vi "Off Mode Standby Mode Power Measure SM.vi"(0 "Power":T3={"Yokogawa"={"WT210"={"Sample Rate (1: 0.25s)"=1, "A Range (12: 20A)"=11, "V Range (6: 600V)"=4, "Power VISA Yokogawa WT210"="WT210"}, "WT500"={"Power VISA Yokogawa WT500"="WT500", "V Range (8: 1000V)"=6, "I Range (7: 40A)"=7, "Update Rate (3: 500ms)"=2}, "WT310_2"={"Sample Rate (1: 0.25s)"=1, "A Range (12: 20A)"=11, "V Range (6: 600V)"=4, "Power VISA Yokogawa WT310_2"=""}, "WT310_3"={"Sample Rate (1: 0.25s)"=1, "A Range (12: 20A)"=11, "V Range (6: 600V)"=4, "Power VISA Yokogawa WT310_3"=""}}, "Aplus"={"Aplus IP Address"="192.168.1.101", "Remote Port"=502, "Instrument"="APLUS", "Instr Driver Revision"="1.03.0053"}, "Power Limits"={"Crest Factor"={"Upper Limit"=1.49, "Lower Limit"=1.34}, "Harmonic Content"={"Uthd"=2.0}, "Voltage"={"% Error"=2.0}, "Stability"={"<1 Watt "={"Wattage"=1.0, "Slope (mW/H)"=10.0}, ">1 Watt"={"1%Power/Hour"=1.0}}}, "Nominal Voltage"=120, "Time Limit (s)"=10800.0, "Power Variation Limit (%)"=50.0, "Power Supply"={"Chroma 61605"="CHROMA", "Use Chroma?"=FALSE}} {"Yokogawa"."WT310_3"."V Range (6: 600V)" items=["Auto", "15V", "30V", "60V", "150V", "300V", "600V"]; "Yokogawa"."WT310_3"."A Range (12: 20A)" items=["Auto", "5mA", "10mA", "20mA", "50mA", "100mA", "200mA", "0.5A", "1A", "2A", "5A", "10A", "20A", "50mV", "100mV", "200mV", "2.5V", "5V", "10V"]; "Yokogawa"."WT310_3"."Sample Rate (1: 0.25s)" items=["0.1s", "0.25s", "0.5s", "1s", "2s", "5s"]; "Yokogawa"."WT310_2"."V Range (6: 600V)" items=["Auto", "15V", "30V", "60V", "150V", "300V", "600V"]; "Yokogawa"."WT310_2"."A Range (12: 20A)" items=["Auto", "5mA", "10mA", "20mA", "50mA", "100mA", "200mA", "0.5A", "1A", "2A", "5A", "10A", "20A", "50mV", "100mV", "200mV", "2.5V", "5V", "10V"]; "Yokogawa"."WT310_2"."Sample Rate (1: 0.25s)" items=["0.1s", "0.25s", "0.5s", "1s", "2s", "5s"]; "Yokogawa"."WT500"."Update Rate (3: 500ms)" items=["-", "100ms", "200ms", "500ms", "1s", "2s", "5s"]; "Yokogawa"."WT500"."I Range (7: 40A)" items=["AUTO", "500 mA", "1 A", "2 A", "5 A", "10 A", "20 A", "40 A", "S-AUTO", "50 mV", "100 mV", "200 mV", "500 mV", "1 V", "2 V", "5 V", "10 V", "250 mA", "500 mA", "1 A", "2.5 A", "5 A", "10 A", "20 A", "25 mV", "50 mV", "100 mV", "250 mV", "500 mV", "1 V", "2.5 V", "5 V"]; "Yokogawa"."WT500"."V Range (8: 1000V)" items=["AUTO", "15", "30", "60", "100", "150", "300", "600", "1000", "7.5", "15", "30", "50", "75", "150", "300", "500"]; "Yokogawa"."WT210"."V Range (6: 600V)" items=["Auto", "15V", "30V", "60V", "150V", "300V", "600V"]; "Yokogawa"."WT210"."A Range (12: 20A)" items=["Auto", "5mA", "10mA", "20mA", "50mA", "100mA", "200mA", "0.5A", "1A", "2A", "5A", "10A", "20A", "50mV", "100mV", "200mV", "2.5V", "5V", "10V"]; "Yokogawa"."WT210"."Sample Rate (1: 0.25s)" items=["0.1s", "0.25s", "0.5s", "1s", "2s", "5s"]}, 1 "Station Label":string="Single Phase 2W", 2 "Appliance Common":T1, 5 "Power Analyzer":T4=enum."APLUS", 11 "Error In":errorcluster) -> (6 "Standby Power Out":T5={"Standby Power Spreadsheet"=[], "Standby Power - Pia (Watts)"=0.0, "Off Mode Power - Poff (Watts)"=0.0, "Sia hr/yr"=8620.0, "Soff hr/yr"=0.0, "Yearly Energy Etso kWh/yr"=0.0, "Maximum Power (Watts)"=0.0, "Power Variation (%)"=0.0, "Slope (mW/hr)"=0.0, "Final Harmonics-U1 (%)"="", "Final Harmonics-U2 (%)"="", "Energy (Wh)"=0.0}, 15 "Error Out":errorcluster)   [LabVIEW 2018]
uses:
  Type Definitions/UTILITY Power Inputs Control.ctl
  Type Definitions/UTILITY Power Analyzer.ctl
  Type Definitions/Standby Power Main Data.ctl
  Custom Pallet Controls/Custom Pallet DBL.ctl
  Washer DOE/Type Definitions/DOE Appliance Common.ctl
  Type Definitions/Standby Power Data Arrays.ctl
  Type Definitions/Standby Power Test Routine.ctl
  Drivers/Yokogawa WT200 Series/Yokogawa WT200 Series.lvlib
panel:
  out "User Notice":string
  out "Description 4":string="Single Phase 2W"
  out "Elapsed Time.":dbl format="%<%H:%M:%S>t"
  in  "Disable Plot":bool
  in  "Pause Graph":bool
  out "XY Graph":T2(graph)
  in  "Y-Axis-2":string(combo)
  in  "Y-Axis-1":string(combo)
  in  "X-Axis":string(combo)
  out "Data":string[][](array[string])
  out "Description":string="IEC 62301 Edition 2.0 2011-01\nHousehold Electrical Appliances - Measurment of standby power"
  in  "Tab Control":enum32{"Input Parameters", "Debug"}(tab)
  in  "Debug":bool
  out "Current State":string
  in  "First 1/3 Timer\n(300 Seconds)":dbl=300.0
  in  "Last 2/3 Timer\n(600 Seconds)":dbl=600.0
  in  "Standby Power In":T5={"Standby Power Spreadsheet"=[], "Standby Power - Pia (Watts)"=0.0, "Off Mode Power - Poff (Watts)"=0.0, "Sia hr/yr"=8620.0, "Soff hr/yr"=0.0, "Yearly Energy Etso kWh/yr"=0.0, "Maximum Power (Watts)"=0.0, "Power Variation (%)"=0.0, "Slope (mW/hr)"=0.0, "Final Harmonics-U1 (%)"="", "Final Harmonics-U2 (%)"="", "Energy (Wh)"=0.0}
  in  "Debug?":bool=TRUE
  out "Debug State":string[](array[string])
  out "Initialization File":string[][](array[string])
  in  "K(0.3)":dbl=0.3 format="%#_13g"
  out "Main Loop Rate":T6 format="%.2f"
  in  "Initialize Rate":bool
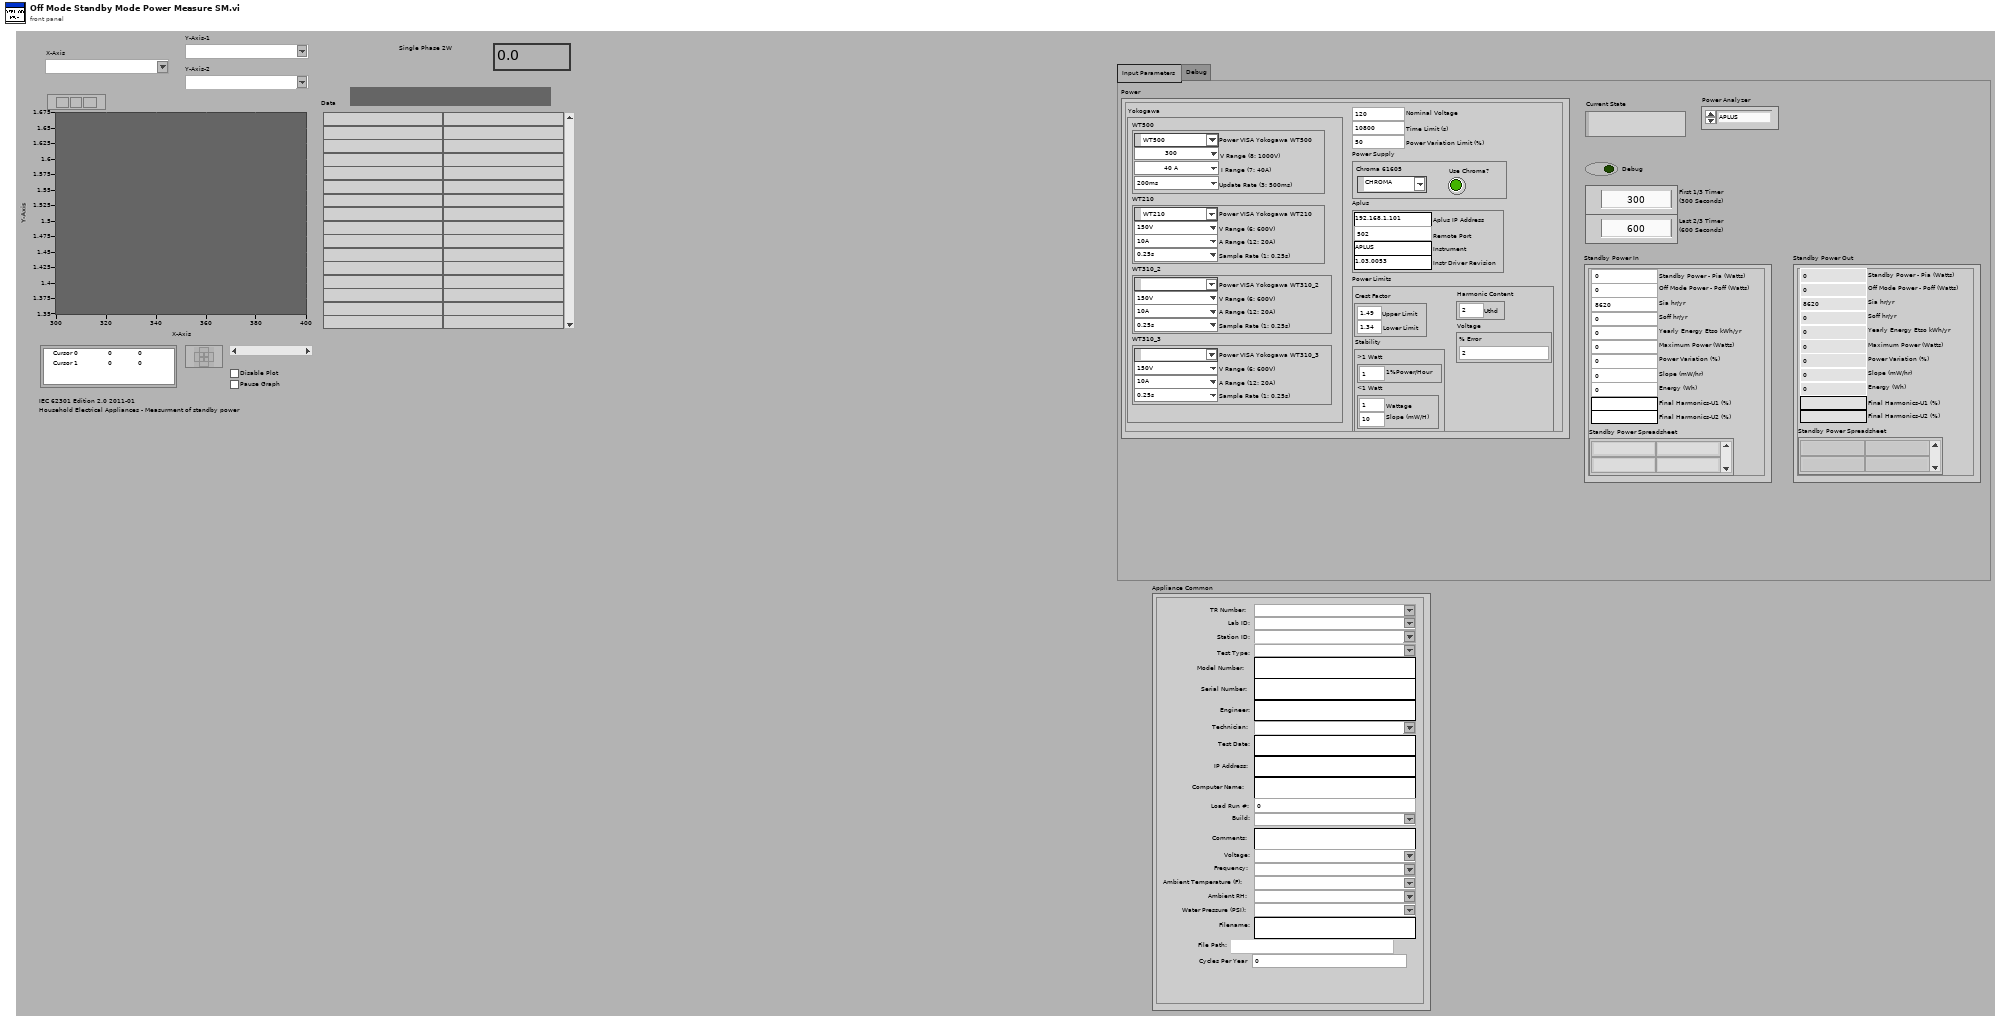
[diagram p1: front panel]
types:
  T1 = typedef "DOE Appliance Common.ctl" = cluster{"Engineer:":string, "Model Number:":string, "Serial Number:":string, "Comments:":string, "Station ID:":string, "Technician:":string, "TR Number:":string, "Lab ID:":string, "Voltage:":string, "Water Pressure (PSI):":string, "Test Date:":string, "Computer Name:":string, "IP Address:":string, "Ambient RH:":string, "Frequency:":string, "Build:":string, "Filename:":string, "Test Type:":string, "Load Run #:":i32, "Ambient Temperature (F):":string, "File Path:":path, "Cycles Per Year":u32}
  T2 = cluster{"Time Array Output":dbl[], "Data Array Output":dbl[]}[]
  T3 = typedef "UTILITY Power Inputs Control.ctl" = cluster{"Yokogawa":cluster{"WT210":cluster{"Sample Rate (1: 0.25s)":i32, "A Range (12: 20A)":i32, "V Range (6: 600V)":i32, "Power VISA Yokogawa WT210":refnum<visa-resource-name>}, "WT500":cluster{"Power VISA Yokogawa WT500":refnum<visa-resource-name>, "V Range (8: 1000V)":i32, "I Range (7: 40A)":i32, "Update Rate (3: 500ms)":i32}, "WT310_2":cluster{"Sample Rate (1: 0.25s)":i32, "A Range (12: 20A)":i32, "V Range (6: 600V)":i32, "Power VISA Yokogawa WT310_2":refnum<visa-resource-name>}, "WT310_3":cluster{"Sample Rate (1: 0.25s)":i32, "A Range (12: 20A)":i32, "V Range (6: 600V)":i32, "Power VISA Yokogawa WT310_3":refnum<visa-resource-name>}}, "Aplus":cluster{"Aplus IP Address":string, "Remote Port":i32, "Instrument":string, "Instr Driver Revision":string}, "Power Limits":cluster{"Crest Factor":cluster{"Upper Limit":dbl, "Lower Limit":dbl}, "Harmonic Content":cluster{"Uthd":dbl}, "Voltage":cluster{"% Error":dbl}, "Stability":cluster{"<1 Watt ":cluster{"Wattage":dbl, "Slope (mW/H)":dbl}, ">1 Watt":cluster{"1%Power/Hour":dbl}}}, "Nominal Voltage":i32, "Time Limit (s)":dbl, "Power Variation Limit (%)":dbl, "Power Supply":cluster{"Chroma 61605":refnum<visa-resource-name>, "Use Chroma?":bool}}
  T4 = typedef "UTILITY Power Analyzer.ctl" = enum16{"", "APLUS", "WT210", "WT500", "WT300", "OSI", "Debug", "WT230", "WT300_1", "WT300_2"}
  T5 = typedef "Standby Power Main Data.ctl" = cluster{"Standby Power Spreadsheet":string[][], "Standby Power - Pia (Watts)":dbl, "Off Mode Power - Poff (Watts)":dbl, "Sia hr/yr":dbl, "Soff hr/yr":dbl, "Yearly Energy Etso kWh/yr":dbl, "Maximum Power (Watts)":dbl, "Power Variation (%)":dbl, "Slope (mW/hr)":dbl, "Final Harmonics-U1 (%)":string, "Final Harmonics-U2 (%)":string, "Energy (Wh)":dbl}
  T6 = typedef "Custom Pallet DBL.ctl" = dbl
  T7 = cluster{"Part 1":bool, "Part 2":bool, "Part 3":bool}
  T8 = enum32{"invalid app kind", "Development System", "Run Time System", "Student Edition", "Embedded LabVIEW", "Evaluation", "Custom"}
  T9 = enum32{"Invalid", "Standard", "Closed", "Hidden", "Minimized", "Maximized"}
  T10 = typedef "Standby Power Data Arrays.ctl" = cluster{"15 Min Data Array":dbl[][], "5 Min Data Array":dbl[][]}
  T11 = typedef "Standby Power Test Routine.ctl" = cluster{"Part 1":bool, "Part 2":bool, "Part 3":bool}
  T12 = cluster{"Core":cluster{"Current VI Reference":refnum<vi>, "Close Panel on Exit?":bool}, "Standby Power Array":T10, "Power ":T3, "Loop Index":i32, "Header File":string[][], "Power Analyzer":T4, "Standby Power In":T5, "Total Array":string[][], "Current State":T11, "Save Data":string[][], "Write Header":bool, "Data Process Timer Reset":bool, "Error?":bool, "Reset Timer?":bool, "Appliance Common":T1}
  T13 = cluster{"Current VI Reference":refnum<vi>, "Close Panel on Exit?":bool}
  T14 = typedef "UTILITY Power Data.ctl" = cluster{"Current (A):Element 1":dbl, "Current (A):Element 2":dbl, "Power (W):Sigma":dbl, "Watt Hours (Wh):Sigma":dbl, "Voltage (V):Element 2":dbl, "Voltage (V):Element 1":dbl, "Current Crest Factor:Element 1":dbl, "Current Crest Factor:Element 2":dbl, "Voltage Harmonic (%):Element 1":dbl, "Voltage Harmonic (%):Element 2":dbl, "Voltage Crest Factor:Element 1":dbl, "Voltage Crest Factor:Element 2":dbl, "Time:Element 1":dbl, "Frequency (Hz):Element 1":dbl, "Apparent Power (VA):Element 1":dbl, "Apparent Power (VA):Element 2":dbl, "Power Factor:Element 1":dbl, "Power Factor:Element 2":dbl, "Max Watt Hours":dbl, "Voltage (V):Element 2 Avg":dbl, "Voltage (V):Element 1 Avg":dbl}
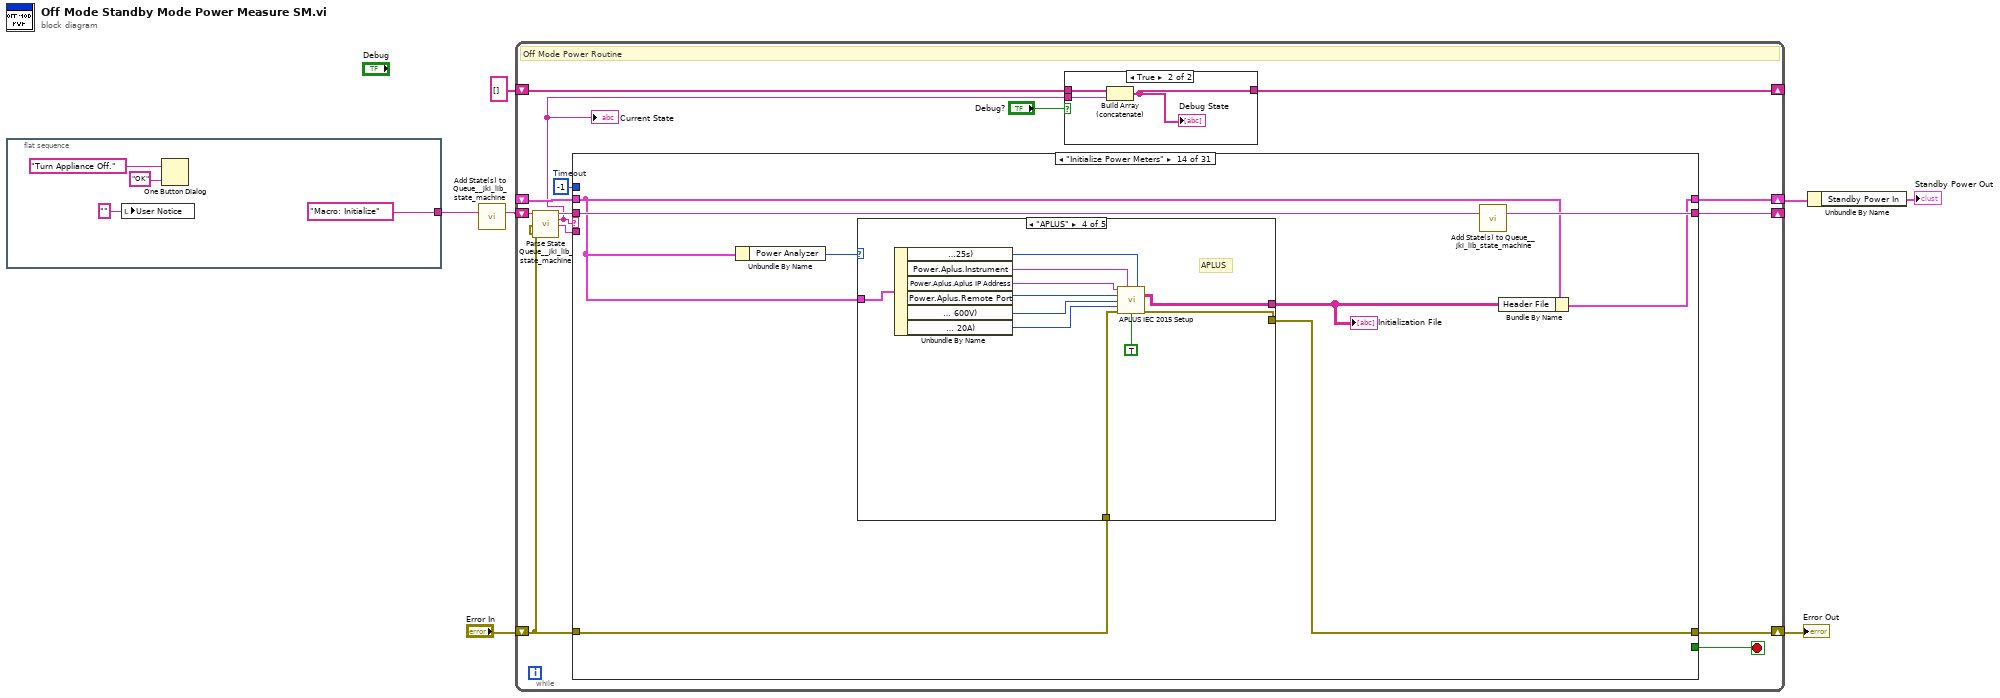
[diagram p0: block diagram]
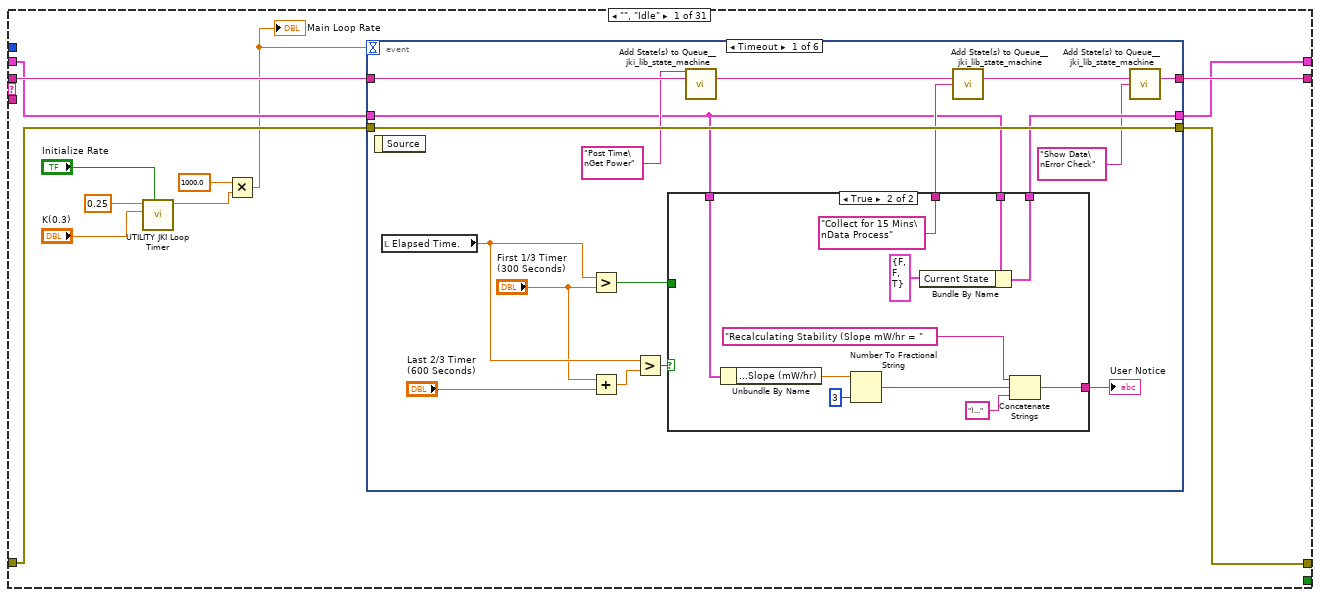
[diagram p3: hidden frame]
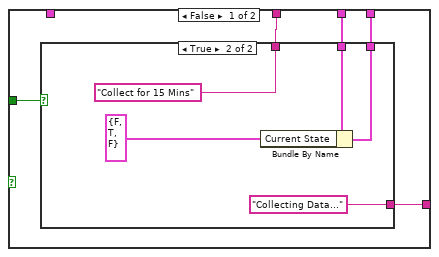
[diagram p4: hidden frame]
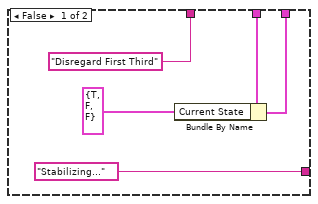
[diagram p5: hidden frame]
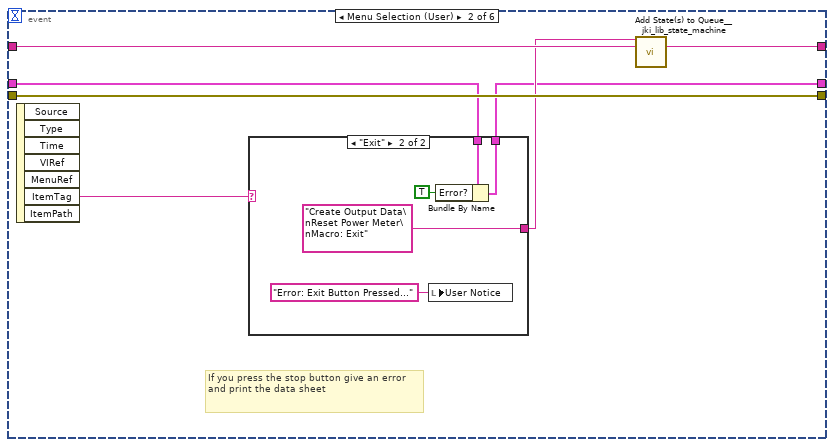
[diagram p6: hidden frame]
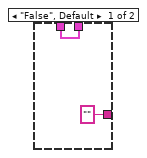
[diagram p7: hidden frame]
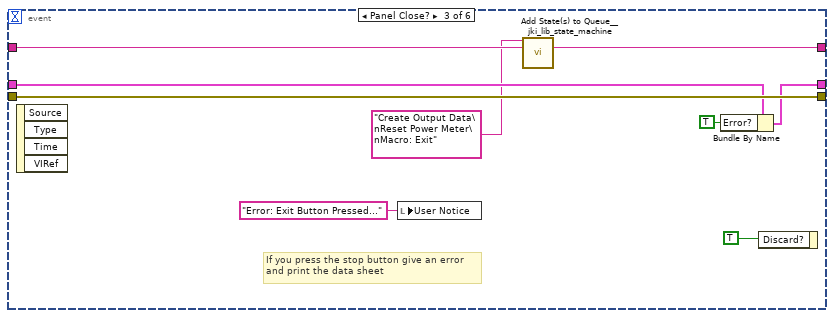
[diagram p8: hidden frame]
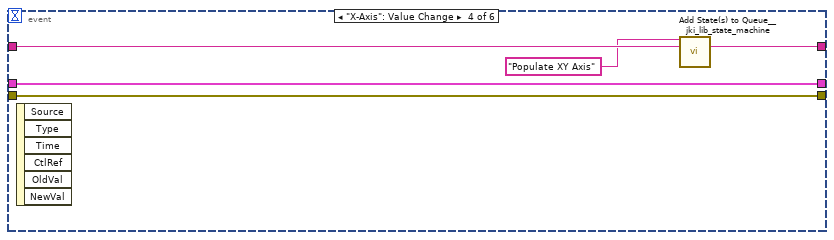
[diagram p9: hidden frame]
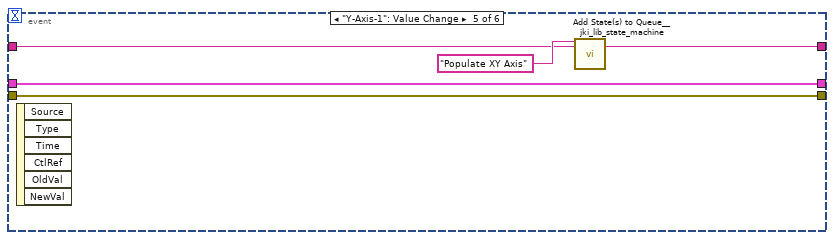
[diagram p10: hidden frame]
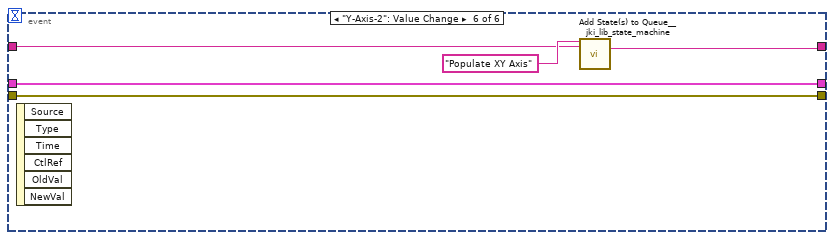
[diagram p11: hidden frame]
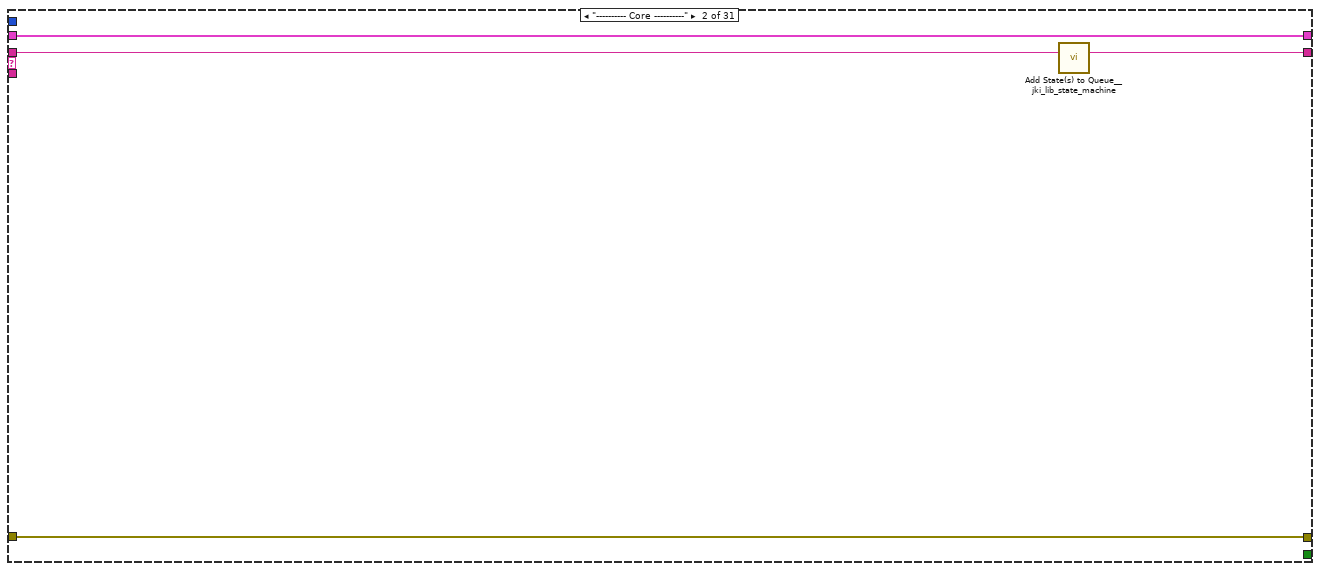
[diagram p12: hidden frame]
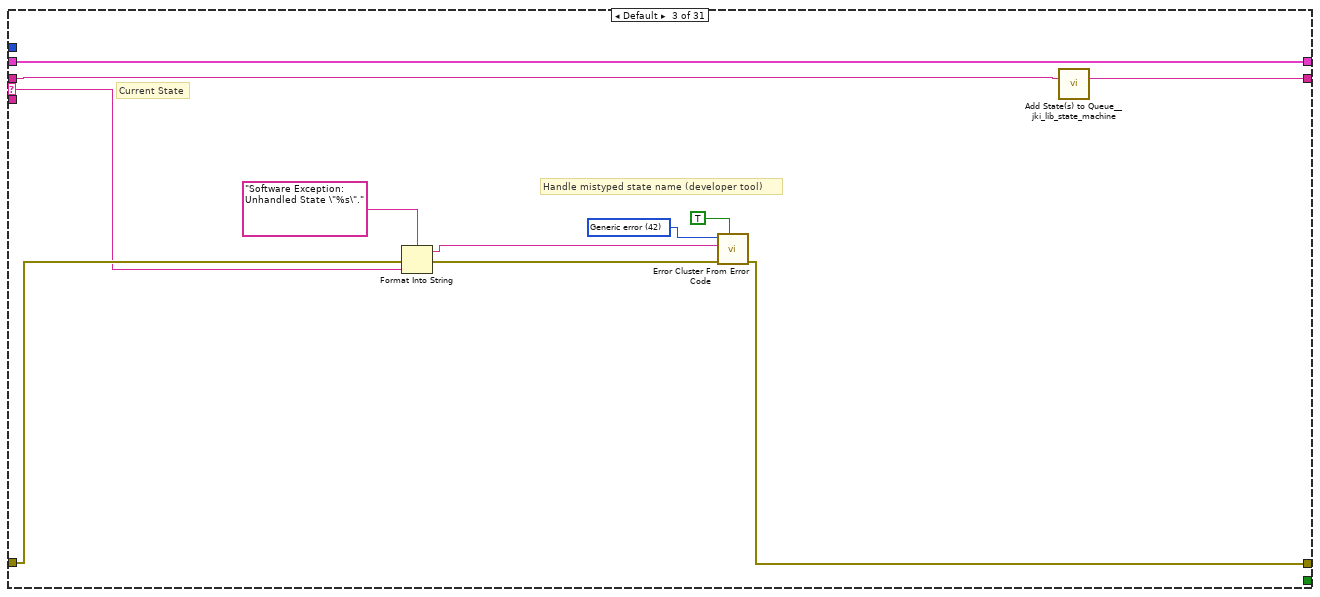
[diagram p13: hidden frame]
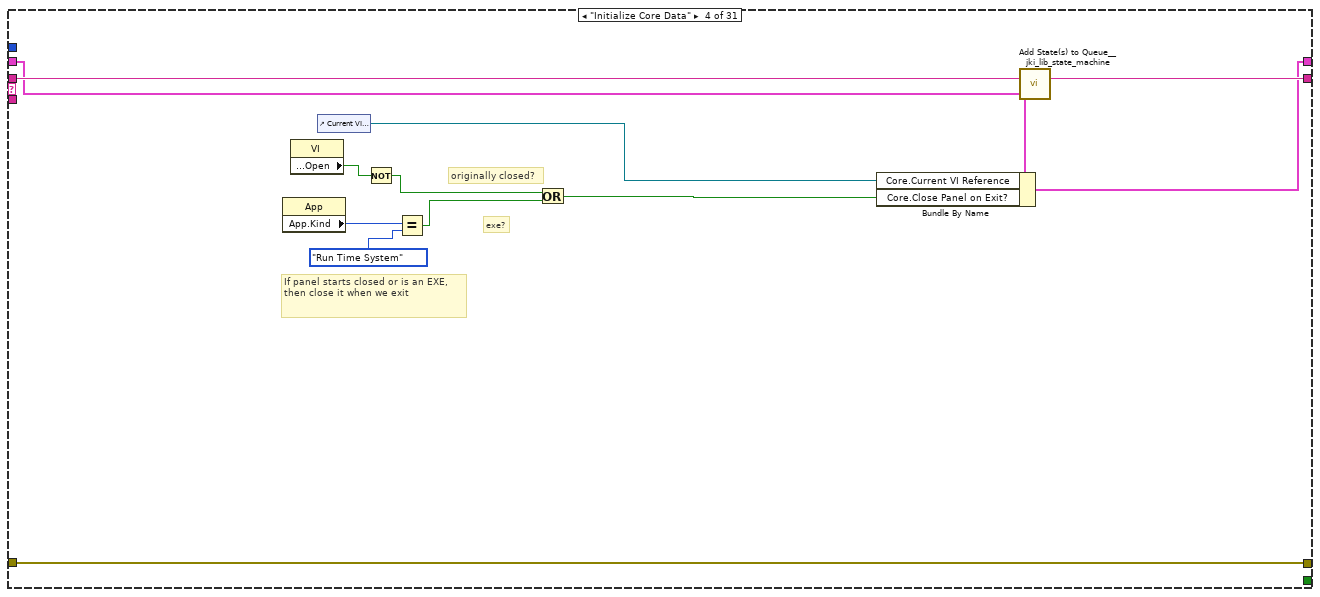
[diagram p14: hidden frame]
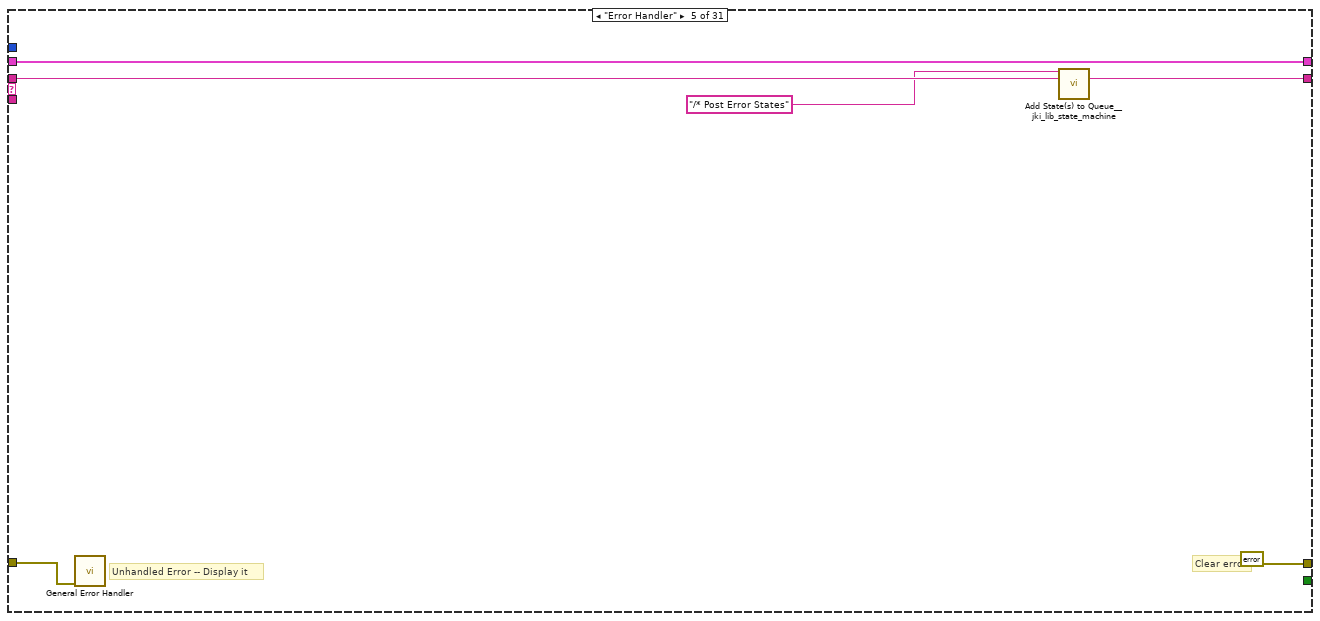
[diagram p15: hidden frame]
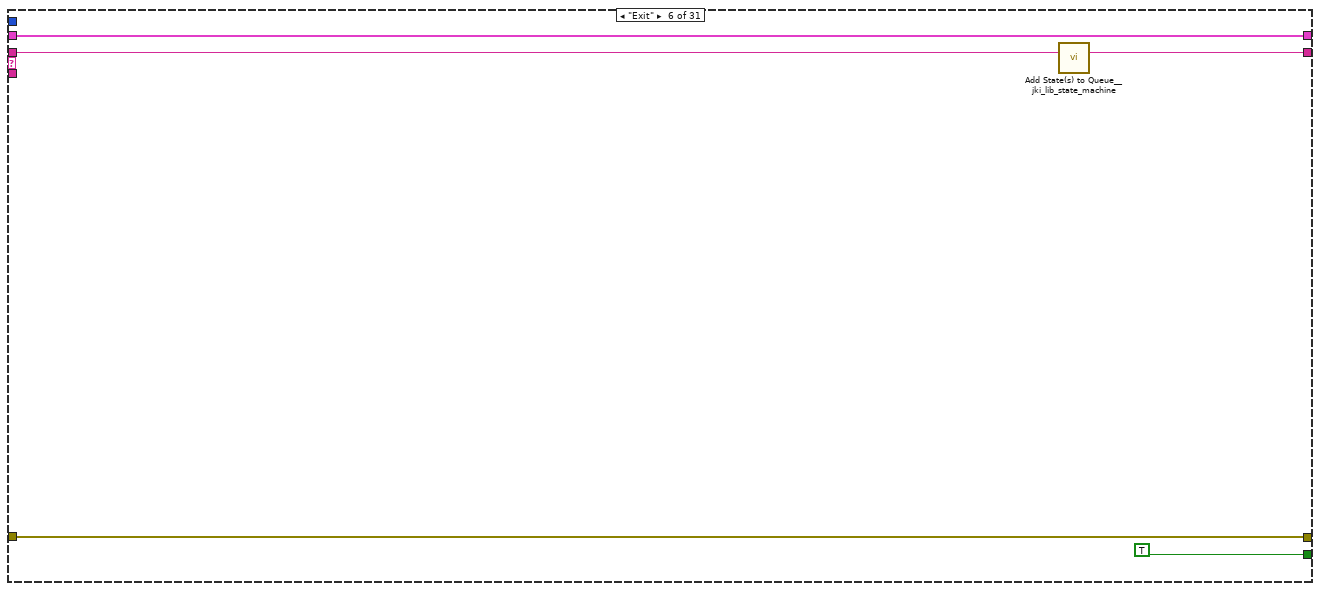
[diagram p16: hidden frame]
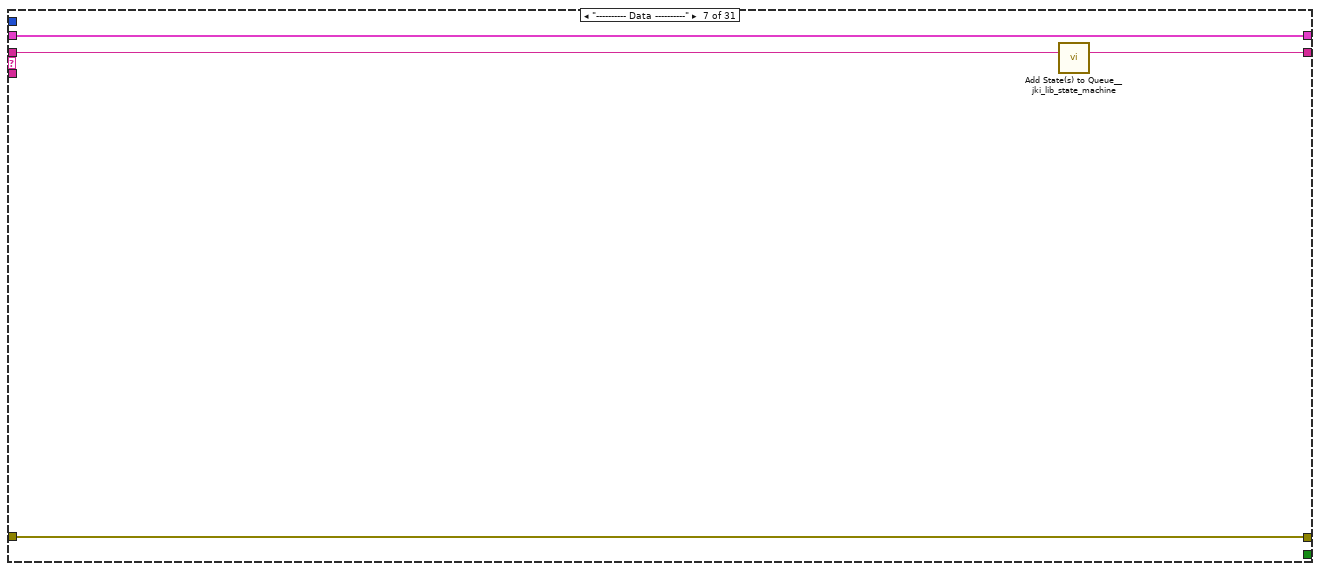
[diagram p17: hidden frame]
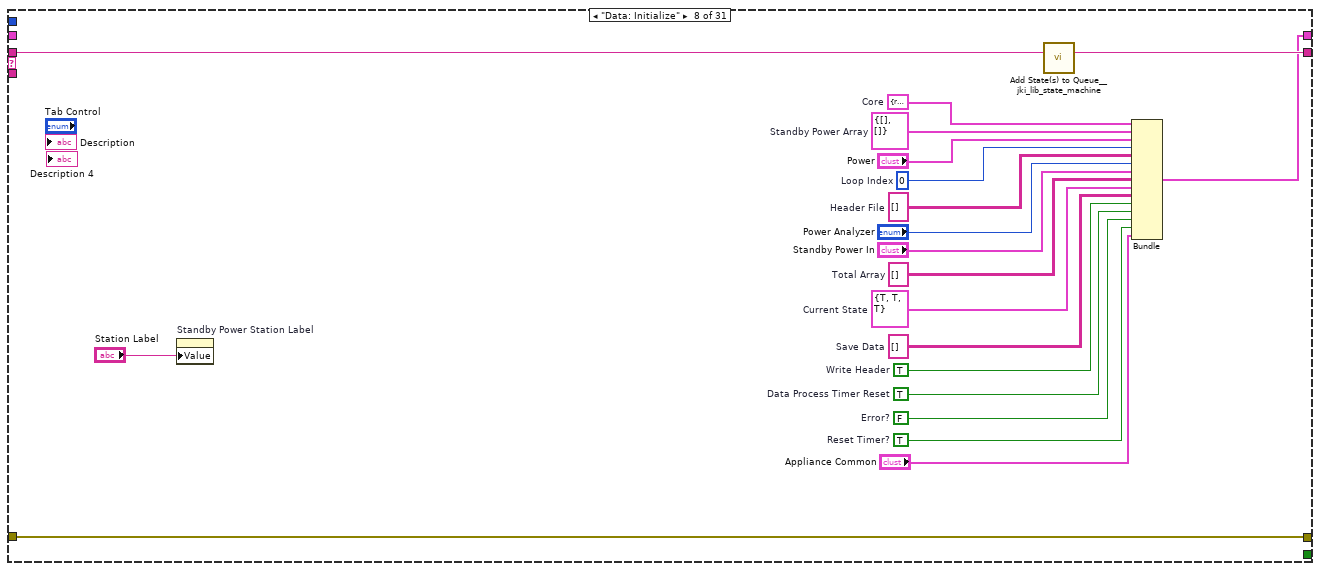
[diagram p18: hidden frame]
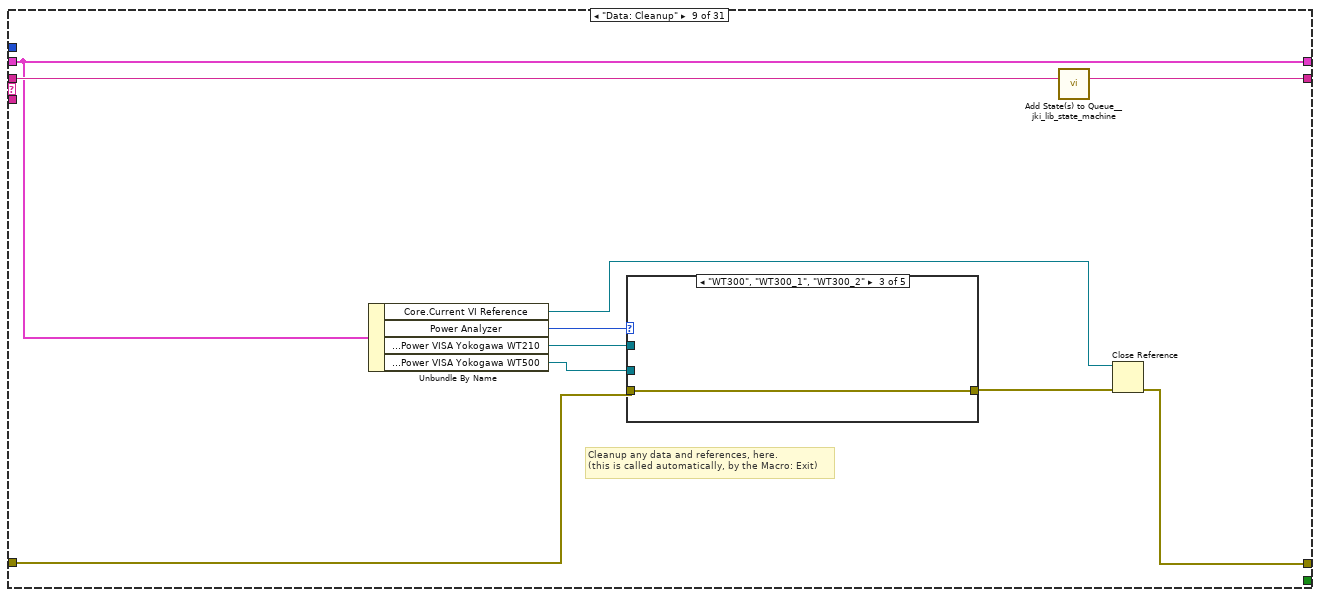
[diagram p19: hidden frame]
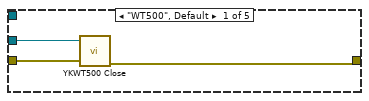
[diagram p20: hidden frame]
diagram:
  n1 = flat-sequence {
    tunnel: ["Macro: Initialize"] -> w1
    frame #0 {
      n2 = local write "User Notice"("" ("User Notice")) -> ()
      n3 = One Button Dialog(message="Turn Appliance Off.", button name ("OK")="OK") -> ()  [unwired: 1 out]
    }
  }
  n4 = call <vilib>:"Add State(s) to Queue__jki_lib_state_machine.vi"("State(s) in (\"\")"=w1) -> ("States Out"=w7:string)  [unwired: 14 in]
  n5 = while "Off Mode Power Routine" {
    shift-right: [w20] -> w3
    shift-left: _ -> [w19]
    shift-right: [w22] -> w5
    shift-left: "Error In" -> [w17]
    shift-right: [w12] -> _
    shift-left: w7 -> [w23]
    shift-right: [w14] -> _
    shift-left: string[] [] -> [w13]
    stop <- w21 stop-if-true
    w18 = -1  # Timeout
    # "Off Mode Power Routine"
    n6 = call <vilib>:"Parse State Queue__jki_lib_state_machine.vi"("State Queue"=w23, "Error In (no error)"=w17) -> ("Remaining States"=w25:string, "Current State"=w15:string, "Arguments"=w24:string)  [unwired: 11 in]
    "Current State" <- w15
    n7 = case shown="\"Initialize Power Meters\"" w15 {
      selector: w15 -> [_ _ w127 _ _ _ _ _ _ _ _ _ _ _ _ _ _ _ _ _ _ _ _ _ _ _ _ _ _ _ _]
      tunnel: w25 -> [w41 w126 w131 w149 w155 w160 w164 w184 w194 w210 w214 w220 w231 w259 w308 w356 w360 w365 w375 w379 w390 w405 w456 w471 w484 w525 w527 w531 w554 w564 w607]
      tunnel: w24 -> [_ _ _ _ _ _ _ _ _ _ _ w215 w225 _ _ _ _ _ _ _ _ _ _ _ _ _ _ _ _ _ _]
      tunnel: w19 -> [w39 w123 w129 w140 w152 w158 w161 _ w191 w207 w212 w218 w227 w252 w303 w352 w357 w362 w372 w376 w388 w399 w454 w465 w478 w519 w528 w534 w553 w559 w606]
      tunnel: [w38 w124 w133 w146 errorcluster {"status"=FALSE, "code"=0, "source"=""} ("error out") w157 w162 w182 w192 w208 w211 w216 w228 w255 w305 w354 w358 w363 w373 w377 w380 w401 w449 w462 w482 w523 w526 w541 w552 w561 w608] -> w22
      tunnel: w17 -> [w37 w124 w132 w146 w151 w157 w162 w182 w189 w208 w211 w217 w229 w256 w306 w354 w358 w363 w373 w377 w386 w402 w452 w463 w482 w520 w526 w542 w552 w562 w605]
      tunnel: [w40 w125 w130 w148 w154 w159 w163 w183 w193 w209 w213 w219 w230 w258 w307 w355 w359 w364 w374 w378 w389 w404 w455 w470 w483 w524 w527 w544 w555 w565 w610] -> w12
      tunnel: [_ _ _ _ _ TRUE _ _ _ _ _ _ _ _ _ _ _ _ _ _ _ _ _ _ _ _ _ _ _ _ _] -> w21
      tunnel: [w36 w123 w129 w147 w152 w158 w161 w180 w191 w207 w212 w218 w227 w257 w303 w352 w357 w362 w372 w376 w387 w403 w453 w464 w477 w518 w528 w533 w553 w558 w596] -> w20
      tunnel: w18 -> [_ _ _ _ _ _ _ _ _ _ _ _ _ _ _ _ _ _ _ _ _ _ _ _ _ _ _ _ _ _ _]
      frame "", "Idle" {
        n8 = call "UTILITY JKI Loop Timer.vi"("Initialize Rate"="Initialize Rate", "K(0.3)"="K(0.3)", "Scan Rate (Seconds)"=0.25 ("Scan Rate (Sec)")) -> ("New Time"=w32:dbl)  [unwired: 7 in, 1 out]
        n9 = Multiply(x=T6 1000.0 ("y"), y=w32) -> (x*y=w31:T6)
        "Main Loop Rate" <- w31
        n10 = event shown="[0] Timeout" {
          selector: _ -> [_ _ _ _ _ _]
          dyn-events: _ -> [_ _ _ _ _ _]
          timeout: w31 -> [_ _ _ _ _ _]
          tunnel: w41 -> [w56 w90 w106 w110 w114 w121]
          tunnel: [w46 w89 w105 w109 w113 w120] -> w40
          tunnel: w39 -> [w42 w86 w101 w112 w117 w118]
          tunnel: [w58 w91 w107 w111 w116 w119] -> w38
          tunnel: w37 -> [w58 w91 w107 w111 w116 w119]
          tunnel: [w48 w85 w100 w112 w117 w118] -> w36
          event Timeout {
            n11 = event-data() -> ()  [unwired: 1 in, 1 out]
            n12 = local read "Elapsed Time."() -> (w51:dbl)
            n13 = Greater?(x=w51, y="First 1/3 Timer\n(300 Seconds)") -> (0:w57:bool)
            n14 = Add(x="First 1/3 Timer\n(300 Seconds)", y="Last 2/3 Timer\n(600 Seconds)") -> (x+y=w52:dbl)
            n15 = Greater?(x=w51, y=w52) -> (0:w50:bool)
            n16 = case shown="True" w50 {
              tunnel: w57 -> [w63 _]
              tunnel: [w62 "Collect for 15 Mins\nData Process" ("State(s) in Front (\"\")")] -> w44
              tunnel: w42 -> [w61 w83]
              tunnel: [w60 w82] -> w48
              tunnel: [w59 w75] -> w43
              tunnel: w42 -> [_ w80]
              frame False {
                n17 = case shown="True" w63 {
                  tunnel: ["Disregard First Third" ("State(s) in Front (\"\")") "Collect for 15 Mins" ("State(s) in Front (\"\")")] -> w62
                  tunnel: w61 -> [w67 w72]
                  tunnel: [w66 w71] -> w60
                  tunnel: ["Stabilizing..." "Collecting Data..."] -> w59
                  frame False {
                    n18 = Bundle By Name(cluster=w67, "Current State"=T7 {"Part 1"=TRUE, "Part 2"=FALSE, "Part 3"=FALSE}) -> (w66:T12)
                  }
                  frame True {
                    n19 = Bundle By Name(cluster=w72, "Current State"=T7 {"Part 1"=FALSE, "Part 2"=TRUE, "Part 3"=FALSE}) -> (w71:T12)
                  }
                }
              }
              frame True {
                n20 = Unbundle By Name(w80) -> ("Standby Power In.Slope (mW/hr)"=w79:dbl)
                n21 = Number To Fractional String(number=w79, precision (6)=i16 3) -> (F-format string=w77:string)  [unwired: 2 in]
                n22 = Bundle By Name(cluster=w83, "Current State"=T7 {"Part 1"=FALSE, "Part 2"=FALSE, "Part 3"=TRUE}) -> (w82:T12)
                n23 = Concatenate Strings("Recalculating Stability (Slope mW/hr = ", w77, ")..." ("string")) -> (w75:string)
              }
            }
            "User Notice" <- w43
            n24 = call <vilib>:"Add State(s) to Queue__jki_lib_state_machine.vi"("State(s) in Front (\"\")"="Post Time\nGet Power" ("State(s) in Front (\"\")"), "State(s) in (\"\")"=w56) -> ("States Out"=w55:string)  [unwired: 13 in]
            n25 = call <vilib>:"Add State(s) to Queue__jki_lib_state_machine.vi"("State(s) in (\"\")"=w55, "State(s) at Back (\"\")"=w44) -> ("States Out"=w47:string)  [unwired: 13 in]
            n26 = call <vilib>:"Add State(s) to Queue__jki_lib_state_machine.vi"("State(s) in (\"\")"=w47, "State(s) at Back (\"\")"="Show Data\nError Check" ("State(s) in Front (\"\")")) -> ("States Out"=w46:string)  [unwired: 13 in]
          }
          event Menu Selection (User) {
            # "If you press the stop button give an error\nand print the data sheet"
            n27 = event-data() -> ("ItemTag"=w88:string)  [unwired: 1 in, 6 out]
            n28 = case shown="\"Exit\"" w88 {
              tunnel: ["" "Create Output Data\nReset Power Meter\nMacro: Exit" ("source")] -> w87
              tunnel: w86 -> [w92 w98]
              tunnel: [w92 w97] -> w85
              frame "False", Default {
              }
              frame "Exit" {
                n29 = local write "User Notice"("Error: Exit Button Pressed...") -> ()
                n30 = Bundle By Name(cluster=w98, "Error?"=TRUE) -> (w97:T12)
              }
            }
            n31 = call <vilib>:"Add State(s) to Queue__jki_lib_state_machine.vi"("State(s) in Front (\"\")"=w87, "State(s) in (\"\")"=w90) -> ("States Out"=w89:string)  [unwired: 13 in]
          }
          event Panel Close? {
            # "If you press the stop button give an error\nand print the data sheet"
            n32 = event-data() -> ()  [unwired: 1 in, 4 out]
            n33 = local write "User Notice"("Error: Exit Button Pressed...") -> ()
            n34 = call <vilib>:"Add State(s) to Queue__jki_lib_state_machine.vi"("State(s) in Front (\"\")"="Create Output Data\nReset Power Meter\nMacro: Exit" ("source"), "State(s) in (\"\")"=w106) -> ("States Out"=w105:string)  [unwired: 13 in]
            n35 = Bundle By Name(cluster=w101, "Error?"=TRUE) -> (w100:T12)
            n36 = event-data("Discard?"=TRUE) -> ()  [unwired: 1 in, 1 out]
          }
          event "X-Axis": Value Change {
            n37 = event-data() -> ()  [unwired: 1 in, 6 out]
            n38 = call <vilib>:"Add State(s) to Queue__jki_lib_state_machine.vi"("State(s) in Front (\"\")"="Populate XY Axis" ("State(s) in Front (\"\")"), "State(s) in (\"\")"=w110) -> ("States Out"=w109:string)  [unwired: 13 in]
          }
          event "Y-Axis-1": Value Change {
            n39 = event-data() -> ()  [unwired: 1 in, 6 out]
            n40 = call <vilib>:"Add State(s) to Queue__jki_lib_state_machine.vi"("State(s) in Front (\"\")"="Populate XY Axis" ("State(s) in Front (\"\")"), "State(s) in (\"\")"=w114) -> ("States Out"=w113:string)  [unwired: 13 in]
          }
          event "Y-Axis-2": Value Change {
            n41 = event-data() -> ()  [unwired: 1 in, 6 out]
            n42 = call <vilib>:"Add State(s) to Queue__jki_lib_state_machine.vi"("State(s) in Front (\"\")"="Populate XY Axis" ("State(s) in Front (\"\")"), "State(s) in (\"\")"=w121) -> ("States Out"=w120:string)  [unwired: 13 in]
          }
        }
      }
      frame "---------- Core ----------" {
        n43 = call <vilib>:"Add State(s) to Queue__jki_lib_state_machine.vi"("State(s) in (\"\")"=w126) -> ("States Out"=w125:string)  [unwired: 14 in]
      }
      frame Default {
        w136 = 42 items=["No error", "Argument error", "Memory is full", "Out of zone", "End of file", "File already open", "Generic file I/O error", "File not found", "File permission error", "Disk is full", "Duplicate path", "Too many files open", "System feature not enabled", "Resource file not found", "Cannot add resource", "Resource not found", "Image not found", "Image memory error", "Pen does not exist", "Config type invalid", "Config token not found", "Config parse error", "Config memory error", "Bad external code format", "Bad external code offset", "External code not present", "Null window", "Destroy window error", "Null menu", "Print aborted", "Bad print record", "Print driver error", "Windows error during printing", "Memory error during printing", "Print dialog error", "Generic print error", "Invalid device refnum", "Device not found", "Device parameter error", "Device unit error", "Cannot open device", "Device call aborted", "Generic error", "Cancelled by user", "Object ID too low", "Object ID too high", "Object not in heap", "Unknown heap", "Unknown object (invalid DefProc)", "Unknown object (DefProc not in table)", "Message out of range", "Invalid (null) method", "Unknown message", "Manager call not supported", "Bad address", "Network operation in progress", "Network operation timed out", "Connection is busy", "Network attribute not supported", "Network error", "Address in use", "System out of memory", "Connection aborted", "Connection refused", "Not connected", "Already connected", "Connection closed", "Initialization error (interapplication manager)", "Bad occurrence", "Wait on unbound occurrence handler", "Occurrence queue overflow", "Datalog type conflict", "Unused", "Unrecognized type (interapplication manager)", "Memory corrupt", "Failed to make temporary DLL", "Old CIN version", "Drag socket not found", "Failed to load drop-object", "Failed to register OLE object", "Failed to release OLE object", "Format specifier type mismatch", "Unknown format specifier", "Too few format specifiers", "Too many format specifiers", "Scan failed", "Newer CIN version", "Error converting to variant", "Runtime menu error", "Password tampered", "Variant attribute not found", "Incompatible variant data type", "Event data is not available", "Event Store is not present", "Occurrence is not found", "Event Queue is not created", "Event info is not available", "Refnum passed is NULL", "Error retrieving Class GUID", "Error retrieving CoClass GUID", "Error retrieving TypeLib GUID.", "Bad built application magic bytes.", "Specific driver is different from the specific driver associated with the Logical Name.", "There is no session opened to the class driver.", "Max Error", "MAX - Error with config objects", "MAX - Error loading configuration", "MAX - Group not supported"]
        # "Current State"
        # "Handle mistyped state name (developer tool)"
        n44 = Format Into String(format string="Software Exception: Unhandled State \"%s\"." ("message"), error in=w132, w127) -> (resulting string=w135:string, error out=w134:errorcluster)  [unwired: 1 in]
        n45 = call <vilib>:"Error Cluster From Error Code.vi"("show call chain? (False)"=TRUE, "error in (no error)"=w134, "error message (\"\")"=w135, "error code (0)"=w136) -> ("error out"=w133:errorcluster)  [unwired: 5 in]
        n46 = call <vilib>:"Add State(s) to Queue__jki_lib_state_machine.vi"("State(s) in (\"\")"=w131) -> ("States Out"=w130:string)  [unwired: 14 in]
      }
      frame "Initialize Core Data" {
        # "originally closed?"
        # "exe?"
        # "If panel starts closed or is an EXE, then close it when we exit"
        n47 = property class="App"() -> ("App.Kind"=w144:T8)  [unwired: 2 in, 2 out]
        n48 = property class="VI"() -> ("Front Panel.Open"=w145:bool)  [unwired: 2 in, 2 out]
        n49 = control-ref of="Current VI Reference"() -> (w138:refnum<vi>)
        n50 = Not(x=w145) -> (.not. x?=w142:bool)
        n51 = Equal?(x=w144, y=T8."Run Time System" ("Application:Kind")) -> (x = y?=w141:bool)
        n52 = Or(x=w142, y=w141) -> (x .or. y?=w139:bool)
        n53 = Bundle By Name(cluster=w140, "Core.Current VI Reference"=w138, "Core.Close Panel on Exit?"=w139) -> (w147:T12)
        n54 = call <vilib>:"Add State(s) to Queue__jki_lib_state_machine.vi"("State(s) in (\"\")"=w149) -> ("States Out"=w148:string)  [unwired: 14 in]
      }
      frame "Error Handler" {
        # "Unhandled Error -- Display it"
        # "Clear error"
        n55 = call <vilib>:"General Error Handler.vi"("error in (no error)"=w151) -> ()  [unwired: 10 in, 5 out]
        n56 = call <vilib>:"Add State(s) to Queue__jki_lib_state_machine.vi"("State(s) in Front (\"\")"="/* Post Error States", "State(s) in (\"\")"=w155) -> ("States Out"=w154:string)  [unwired: 13 in]
      }
      frame "Exit" {
        n57 = call <vilib>:"Add State(s) to Queue__jki_lib_state_machine.vi"("State(s) in (\"\")"=w160) -> ("States Out"=w159:string)  [unwired: 14 in]
      }
      frame "---------- Data ----------" {
        n58 = call <vilib>:"Add State(s) to Queue__jki_lib_state_machine.vi"("State(s) in (\"\")"=w164) -> ("States Out"=w163:string)  [unwired: 14 in]
      }
      frame "Data: Initialize" {
        w166 = TRUE  # Reset Timer?
        w167 = FALSE  # Error?
        w168 = TRUE  # Data Process Timer Reset
        w169 = TRUE  # Write Header
        w170 = string[][] []  # Save Data
        w171 = T11 {"Part 1"=TRUE, "Part 2"=TRUE, "Part 3"=TRUE}  # Current State
        w172 = string[][] []  # Total Array
        w173 = T10 {"15 Min Data Array"=[], "5 Min Data Array"=[]}  # Standby Power Array
        w177 = string[][] []  # Header File
        w178 = 0  # Loop Index
        w181 = T13 {"Current VI Reference"=refnum, "Close Panel on Exit?"=FALSE}  # Core
        n59 = property on="Standby Power Station Label" class="Str"("Value"="Station Label") -> ()  [unwired: 2 in, 2 out]
        n60 = call <vilib>:"Add State(s) to Queue__jki_lib_state_machine.vi"("State(s) in (\"\")"=w184) -> ("States Out"=w183:string)  [unwired: 14 in]
        n61 = Bundle("Core"=w181, "Standby Power Array"=w173, "Power"="Power", "Loop Index"=w178, "Header File"=w177, "Power Analyzer"="Power Analyzer", "Standby Power In"="Standby Power In", "Total Array"=w172, "Current State"=w171, "Save Data"=w170, "Write Header"=w169, "Data Process Timer Reset"=w168, "Error?"=w167, "Reset Timer?"=w166, "Appliance Common"="Appliance Common") -> (w180:T12)  [unwired: 1 in]
      }
      frame "Data: Cleanup" {
        # "Cleanup any data and references, here.\n(this is called automatically, by the Macro: Exit)"
        n62 = Unbundle By Name(w191) -> ("Core.Current VI Reference"=w185:refnum<vi>, "Power Analyzer"=w187:T4, "Power.Yokogawa.WT210.Power VISA Yokogawa WT210"=w188:refnum<visa-resource-name>, "Power.Yokogawa.WT500.Power VISA Yokogawa WT500"=w186:refnum<visa-resource-name>)
        n63 = case shown="\"WT300\", \"WT300_1\", \"WT300_2\"" w187 {
          tunnel: [w195 w203 w204 w205 w206] -> w190
          tunnel: w189 -> [w196 w201 w204 w205 w206]
          tunnel: w188 -> [_ w199 _ _ _]
          tunnel: w186 -> [w197 _ _ _ _]
          frame "WT500", Default {
            n64 = call "YKWT500 Close.vi"("error in (no error)"=w196, "VISA resource name"=w197) -> ("error out"=w195:errorcluster)  [unwired: 9 in]
          }
          frame "WT210", "WT230" {
            n65 = call "Start Stop Integration.vi"("VISA resource name"=w199, "Start/Stop (F: Stop)"=FALSE, "error in (no error)"=w201) -> ("VISA resource name out"=w198:refnum<visa-resource-name>, "error out"=w200:errorcluster)  [unwired: 11 in]
            n66 = call "Close.vi"("VISA resource name"=w198, "error in (no error)"=w200) -> ("error out"=w203:errorcluster)  [unwired: 13 in]
          }
          frame "WT300", "WT300_1", "WT300_2" {
          }
          frame "Debug" {
          }
          frame "APLUS" {
          }
        }
        n67 = call <vilib>:"Add State(s) to Queue__jki_lib_state_machine.vi"("State(s) in (\"\")"=w194) -> ("States Out"=w193:string)  [unwired: 14 in]
        n68 = Close Reference(reference=w185, error in (no error)=w190) -> (error out=w192:errorcluster)
      }
      frame "---------- UI ----------" {
        n69 = call <vilib>:"Add State(s) to Queue__jki_lib_state_machine.vi"("State(s) in (\"\")"=w210) -> ("States Out"=w209:string)  [unwired: 14 in]
      }
      frame "UI: Initialize" {
        n70 = call <vilib>:"Add State(s) to Queue__jki_lib_state_machine.vi"("State(s) in (\"\")"=w214) -> ("States Out"=w213:string)  [unwired: 14 in]
      }
      frame "UI: Cursor Set" {
        # "Argument"
        n71 = case shown="\"Idle\", Default" w215 {
          tunnel: w217 -> [w222 w224]
          tunnel: [w221 w223] -> w216
          frame "Idle", Default {
            n72 = call <vilib>:"Unset Busy.vi"("error in (no error)"=w222) -> ("error out"=w221:errorcluster)  [unwired: 10 in]
          }
          frame "Busy" {
            n73 = call <vilib>:"Set Busy.vi"("error in (no error)"=w224) -> ("error out"=w223:errorcluster)  [unwired: 9 in, 1 out]
          }
        }
        n74 = call <vilib>:"Add State(s) to Queue__jki_lib_state_machine.vi"("State(s) in (\"\")"=w220) -> ("States Out"=w219:string)  [unwired: 14 in]
      }
      frame "UI: Front Panel State" {
        # "Argument"
        n75 = Unbundle By Name(w227) -> ("Core.Current VI Reference"=w226:refnum<vi>)
        n76 = case shown="\"Open\", Default" w225 {
          tunnel: w229 -> [w235 w248]
          tunnel: [w237 w249] -> w228
          tunnel: w226 -> [w236 w246]
          frame "Open", Default {
            n77 = property class="VI"(reference=w236, error in=w235) -> (reference out=w233:refnum<vi>, error out=w234:errorcluster, "Front Panel.Open"=w232:bool)
            n78 = case shown="True" w232 {
              tunnel: [w240 w243] -> w237
              tunnel: w234 -> [w239 w243]
              tunnel: w233 -> [w238 _]
              frame False {
                n79 = invoke class="VI" method="FP.Open"(reference=w238, error in=w239, "Activate"=TRUE, "State"=T9."Standard") -> (error out=w240:errorcluster)  [unwired: 1 in, 4 out]
              }
              frame True {
              }
            }
          }
          frame "Close" {
            n80 = property class="VI"(reference=w246, error in=w248) -> (reference out=w245:refnum<vi>, error out=w247:errorcluster, "Front Panel.Open"=w244:bool)
            n81 = case shown="True" w244 {
              tunnel: [w250 w251] -> w249
              tunnel: w247 -> [w250 w251]
              tunnel: w245 -> [_ _]
              frame False {
              }
              frame True {
              }
            }
          }
        }
        n82 = call <vilib>:"Add State(s) to Queue__jki_lib_state_machine.vi"("State(s) in (\"\")"=w231) -> ("States Out"=w230:string)  [unwired: 14 in]
      }
      frame "Initialize Power Meters" {
        n83 = Unbundle By Name(w252) -> ("Power Analyzer"=w254:T4)
        n84 = case shown="\"APLUS\"" w254 {
          selector: w254 -> [w260 _ _ _ _]
          tunnel: w256 -> [w267 w280 w289 w300 w302]
          tunnel: [w266 w280 w288 w299 w302] -> w255
          tunnel: [w265 w279 w287 w297 string[][] [["Test", "Test"], ["Test", "Test"]] ("Header File")] -> w253
          tunnel: w252 -> [w264 w278 w284 w296 _]
          frame "WT300", Default {
            # "Default"
            n85 = case shown="\"WT300_2\"" w260 {
              tunnel: w264 -> [w269 w271 w273]
              tunnel: [w268 w270 w272] -> w263
              frame "WT300_1" {
                n86 = Unbundle By Name(w269) -> ("Power.Yokogawa.WT310_2.Power VISA Yokogawa WT310_2"=w268:refnum<visa-resource-name>)
              }
              frame "WT300_2" {
                n87 = Unbundle By Name(w271) -> ("Power.Yokogawa.WT310_3.Power VISA Yokogawa WT310_3"=w270:refnum<visa-resource-name>)
              }
              frame "WT300", Default {
                n88 = Unbundle By Name(w273) -> ("Power.Yokogawa.WT210.Power VISA Yokogawa WT210"=w272:refnum<visa-resource-name>)
              }
            }
            n89 = call "WT300 IEC 2015 Setup.vi"("VISA Input"=w263, "Range Configuration (True)"=bool[] [FALSE, FALSE, FALSE, FALSE, TRUE, TRUE, TRUE, TRUE, FALSE, FALSE, FALSE, FALSE, FALSE], "error in (no error)"=w267, "Enable Auto Range (F: Disable)"=TRUE) -> ("Header File"=w265:string[][], "error out"=w266:errorcluster)  [unwired: 8 in, 2 out]
          }
          frame "WT210", "WT230" {
            # "WT210"
            n90 = Unbundle By Name(w278) -> ("Power.Yokogawa.WT210.Power VISA Yokogawa WT210"=w277:refnum<visa-resource-name>, "Power.Yokogawa.WT210.V Range (6: 600V)"=w274:i32, "Power.Yokogawa.WT210.A Range (12: 20A)"=w275:i32, "Power.Yokogawa.WT210.Sample Rate (1: 0.25s)"=w276:i32)
            n91 = call "WT210 IEC 2015 Setup.vi"("VISA Input"=w277, "V Range (6: 600V)"=w274, "A Range (12: 20A)"=w275, "Sample Rate (1: 0.25s)"=w276) -> ("Header File"=w279:string[][])  [unwired: 8 in, 3 out]
          }
          frame "WT500" {
            w281 = u16 0 items=["AUTO", "15", "30", "60", "100", "150", "300", "600", "1000", "7.5", "15", "30", "50", "75", "150", "300", "500"] ("V Range (8: 1000V)")
            w285 = u16 0 items=["AUTO", "500 mA", "1 A", "2 A", "5 A", "10 A", "20 A", "40 A", "S-AUTO", "50 mV", "100 mV", "200 mV", "500 mV", "1 V", "2 V", "5 V", "10 V", "250 mA", "500 mA", "1 A", "2.5 A", "5 A", "10 A", "20 A", "25 mV", "50 mV", "100 mV", "250 mV", "500 mV", "1 V", "2.5 V", "5 V"] ("I Range (7: 40A)")
            w286 = u16 2 items=["-", "100ms", "200ms", "500ms", "1s", "2s", "5s"] ("Update Rate (3: 500ms)")
            # "WT500"
            n92 = Unbundle By Name(w284) -> ("Power.Yokogawa.WT500.Power VISA Yokogawa WT500"=w283:refnum<visa-resource-name>)
            n93 = call "WT500 IEC 2015 Setup.vi"("VISA Input"=w283, "V Range (8: 1000V)"=w281, "I Range (7: 40A)"=w285, "Update Rate (3: 500ms)"=w286, "Error In"=w289, "Start/Stop (False: Stop)"=FALSE) -> ("Standby Power Header"=w287:string[][], "Error Out"=w288:errorcluster)  [unwired: 5 in, 3 out]
          }
          frame "APLUS" {
            # "APLUS"
            n94 = Unbundle By Name(w296) -> ("Power.Yokogawa.WT210.Sample Rate (1: 0.25s)"=w290:i32, "Power.Aplus.Instrument"=w295:string, "Power.Aplus.Aplus IP Address"=w294:string, "Power.Aplus.Remote Port"=w293:i32, "Power.Yokogawa.WT210.V Range (6: 600V)"=w292:i32, "Power.Yokogawa.WT210.A Range (12: 20A)"=w291:i32)
            n95 = call "APLUS IEC 2015 Setup.vi"("Remote IP Address"=w294, "Instrument"=w295, "Sample Rate (1: 0.25s)"=w290, "Remote Port"=w293, "V Range (6: 600V)"=w292, "A Range (12: 20A)"=w291, "error in"=w300, "Reset WattHours"=TRUE) -> ("Header File"=w297:string[][], "error out"=w299:errorcluster)  [unwired: 5 in, 1 out]
          }
          frame "Debug" {
            # "Debug"
          }
        }
        "Initialization File" <- w253
        n96 = call <vilib>:"Add State(s) to Queue__jki_lib_state_machine.vi"("State(s) in (\"\")"=w259) -> ("States Out"=w258:string)  [unwired: 14 in]
        n97 = Bundle By Name(cluster=w252, "Header File"=w253) -> (w257:T12)
      }
      frame "Reset Power Meter" {
        n98 = Unbundle By Name(w303) -> ("Power Analyzer"=w304:T4)
        n99 = case shown="\"APLUS\"" w304 {
          selector: w304 -> [w309 _ _ _ _]
          tunnel: w306 -> [w313 w321 w334 w344 w345]
          tunnel: [w312 w320 w333 w343 w345] -> w305
          tunnel: w303 -> [w311 w326 w332 w341 _]
          frame "WT300", Default {
            # "Default"
            n100 = case shown="\"WT300_2\"" w309 {
              tunnel: w311 -> [w315 w317 w319]
              tunnel: [w314 w316 w318] -> w310
              frame "WT300_1" {
                n101 = Unbundle By Name(w315) -> ("Power.Yokogawa.WT310_2.Power VISA Yokogawa WT310_2"=w314:refnum<visa-resource-name>)
              }
              frame "WT300_2" {
                n102 = Unbundle By Name(w317) -> ("Power.Yokogawa.WT310_3.Power VISA Yokogawa WT310_3"=w316:refnum<visa-resource-name>)
              }
              frame "WT300", Default {
                n103 = Unbundle By Name(w319) -> ("Power.Yokogawa.WT210.Power VISA Yokogawa WT210"=w318:refnum<visa-resource-name>)
              }
            }
            n104 = call "WT300 IEC 2015 Setup.vi"("VISA Input"=w310, "error in (no error)"=w313) -> ("error out"=w312:errorcluster)  [unwired: 10 in, 3 out]
          }
          frame "WT210", "WT230" {
            # "WT210"
            n105 = Unbundle By Name(w326) -> ("Power.Yokogawa.WT210.Power VISA Yokogawa WT210"=w325:refnum<visa-resource-name>, "Power.Yokogawa.WT210.V Range (6: 600V)"=w322:i32, "Power.Yokogawa.WT210.A Range (12: 20A)"=w323:i32, "Power.Yokogawa.WT210.Sample Rate (1: 0.25s)"=w324:i32)
            n106 = call "WT210 IEC 2015 Setup.vi"("VISA Input"=w325, "V Range (6: 600V)"=w322, "A Range (12: 20A)"=w323, "Sample Rate (1: 0.25s)"=w324, "error in (no error)"=w321) -> ("error out"=w320:errorcluster)  [unwired: 7 in, 3 out]
          }
          frame "WT500" {
            # "WT500"
            n107 = Unbundle By Name(w332) -> ("Power.Yokogawa.WT500.Power VISA Yokogawa WT500"=w331:refnum<visa-resource-name>, "Power.Yokogawa.WT500.V Range (8: 1000V)"=w330:i32, "Power.Yokogawa.WT500.I Range (7: 40A)"=w329:i32, "Power.Yokogawa.WT500.Update Rate (3: 500ms)"=w328:i32)
            n108 = call "WT500 IEC 2015 Setup.vi"("VISA Input"=w331, "V Range (8: 1000V)"=w330, "I Range (7: 40A)"=w329, "Update Rate (3: 500ms)"=w328, "Error In"=w334, "Start/Stop (False: Stop)"=TRUE) -> ("Error Out"=w333:errorcluster)  [unwired: 5 in, 4 out]
          }
          frame "APLUS" {
            # "APLUS"
            n109 = Unbundle By Name(w341) -> ("Power.Yokogawa.WT210.Sample Rate (1: 0.25s)"=w335:i32, "Power.Aplus.Instrument"=w340:string, "Power.Aplus.Aplus IP Address"=w339:string, "Power.Aplus.Remote Port"=w338:i32, "Power.Yokogawa.WT210.V Range (6: 600V)"=w337:i32, "Power.Yokogawa.WT210.A Range (12: 20A)"=w336:i32)
            n110 = call "APLUS IEC 2015 Setup.vi"("Remote IP Address"=w339, "Instrument"=w340, "Sample Rate (1: 0.25s)"=w335, "Remote Port"=w338, "V Range (6: 600V)"=w337, "A Range (12: 20A)"=w336, "error in"=w344, "Reset WattHours"=TRUE) -> ("error out"=w343:errorcluster)  [unwired: 5 in, 2 out]
          }
          frame "Debug" {
            # "Debug"
          }
        }
        n111 = call <vilib>:"Add State(s) to Queue__jki_lib_state_machine.vi"("State(s) in (\"\")"=w308) -> ("States Out"=w307:string)  [unwired: 14 in]
      }
      frame "Populate XY Axis" {
        n112 = Unbundle By Name(w352) -> ("Total Array"=w353:string[][])
        n113 = Index Array(array=w353, index (col)=0 ("disabled index (col)")) -> (element=w351:string[])  [unwired: 1 in]
        n114 = Index Array(array=w353, index (col)=0 ("disabled index (col)")) -> (element=w350:string[])  [unwired: 1 in]
        n115 = Index Array(array=w353, index (col)=0 ("disabled index (col)")) -> (element=w349:string[])  [unwired: 1 in]
        n116 = property on="X-Axis" class="CmbBox"("Strings[]"=w351) -> ()  [unwired: 2 in, 2 out]
        n117 = property on="Y-Axis-1" class="CmbBox"("Strings[]"=w350) -> ()  [unwired: 2 in, 2 out]
        n118 = property on="Y-Axis-2" class="CmbBox"("Strings[]"=w349) -> ()  [unwired: 2 in, 2 out]
        n119 = call <vilib>:"Add State(s) to Queue__jki_lib_state_machine.vi"("State(s) in (\"\")"=w356) -> ("States Out"=w355:string)  [unwired: 14 in]
      }
      frame "---------- Macro ----------" {
        n120 = call <vilib>:"Add State(s) to Queue__jki_lib_state_machine.vi"("State(s) in (\"\")"=w360) -> ("States Out"=w359:string)  [unwired: 14 in]
      }
      frame "Macro: Initialize" {
        w361 = "Data: Initialize\nInitialize Power Meters\nInitialize Core Data\nUI: Initialize\nUI: Front Panel State >> Open\nPost Time\nGet Power\nDisregard First Third\nShow Data\nError Check\nPopulate XY Axis"  # Data: Initialize Initialize Power Meters Initialize Core Data UI: Initialize UI: Front Panel State >> Open Post Time Get Power Disregard First Third Show Data Error Check Populate XY Axis
        n121 = call <vilib>:"Add State(s) to Queue__jki_lib_state_machine.vi"("State(s) in Front (\"\")"=w361, "State(s) in (\"\")"=w365) -> ("States Out"=w364:string)  [unwired: 13 in]
      }
      frame "Macro: Exit" {
        n122 = Unbundle By Name(w372) -> ("Core.Close Panel on Exit?"=w371:bool)
        n123 = Select(t="UI: Front Panel State >> Close", s=w371, f="") -> (s? t:f=w368:string)
        n124 = call <vilib>:"Add State(s) to Queue__jki_lib_state_machine.vi"("State(s) in (\"\")"=w368, "State(s) at Back (\"\")"="Data: Cleanup\nExit") -> ("States Out"=w366:string)  [unwired: 13 in]
        n125 = call <vilib>:"Add State(s) to Queue__jki_lib_state_machine.vi"("State(s) in Front (\"\")"=w366, "State(s) in (\"\")"=w375) -> ("States Out"=w374:string)  [unwired: 13 in]
      }
      frame "------Collect Data ------" {
        n126 = call <vilib>:"Add State(s) to Queue__jki_lib_state_machine.vi"("State(s) in (\"\")"=w379) -> ("States Out"=w378:string)  [unwired: 14 in]
      }
      frame "Post Time" {
        n127 = Unbundle By Name(w388) -> ("Reset Timer?"=w382:bool)
        n128 = call "UTILITY Elapsed Time.vi"("Add Elapsed Time (hrs)"=TRUE, "error in (no error)"=w386, "Reset Timer"=w382) -> ("error out"=w381:errorcluster, "Elapsed Time"=→"Elapsed Time.":dbl, "Total Array"=w385:string[][])  [unwired: 4 in, 2 out]
        n129 = flat-sequence {
          tunnel: w388 -> [w395]
          tunnel: [w394] -> w387
          tunnel: w385 -> [w393]
          tunnel: w381 -> [w391]
          tunnel: [w391] -> w380
          frame #0 {
            n130 = Bundle By Name(cluster=w395, "Reset Timer?"=FALSE, "Total Array"=w393) -> (w394:T12)
          }
        }
        n131 = call <vilib>:"Add State(s) to Queue__jki_lib_state_machine.vi"("State(s) in (\"\")"=w390) -> ("States Out"=w389:string)  [unwired: 14 in]
      }
      frame "Get Power" {
        n132 = Unbundle By Name(w399) -> ("Total Array"=w398:string[][], "Power Analyzer"=w400:T4)
        n133 = case shown="\"WT300\", Default" w400 {
          selector: w400 -> [w408 _ _ _ _ _]
          tunnel: w402 -> [w411 w422 w429 w434 w440 w442]
          tunnel: [w410 w421 w428 w433 w439 w442] -> w401
          tunnel: [w409 w420 w426 w432 w438 string[][] [["Voltage (V) Element 1", "0.000"], ["Voltage (V) Element 2", "236.200"], ["Power (Watts)", "1.52"], ["Current (Amps) Element 1", "236.200"], ["Current (Amps) Element 2", "0.5"], ["Energy (WH)", "0.000"], ["Current Crest Factor Element 1", "0.000"], ["Current Crest Factor Element 2", "0.000"], ["Total Harmonic Distortion (%) Element 1", "0.000"], ["Total Harmonic Distortion (%) Element 2", "0.000"], ["Voltage Crest Factor Element 1", "0.000"], ["Voltage Crest Factor Element 2", "0.000"], ["Integration Timer (sec)", "0.000"], ["Frequency (Hz)", "0.000"], ["Apparent Power (VA) Element 1", "0.000"], ["Apparent Power (VA) Element 2", "0.000"], ["Power Factor Element 1", "0.000"], ["Power Factor Element 2", "0.000"]] ("Data Array")] -> w397
          tunnel: w399 -> [w407 w419 w425 w431 w437 _]
          frame "WT300", Default {
            n134 = case shown="\"WT300\", Default" w408 {
              tunnel: w407 -> [w413 w415 w417]
              tunnel: [w412 w414 w416] -> w406
              frame "WT300_1" {
                n135 = Unbundle By Name(w413) -> ("Power.Yokogawa.WT310_2.Power VISA Yokogawa WT310_2"=w412:refnum<visa-resource-name>)
              }
              frame "WT300_2" {
                n136 = Unbundle By Name(w415) -> ("Power.Yokogawa.WT310_3.Power VISA Yokogawa WT310_3"=w414:refnum<visa-resource-name>)
              }
              frame "WT300", Default {
                n137 = Unbundle By Name(w417) -> ("Power.Yokogawa.WT210.Power VISA Yokogawa WT210"=w416:refnum<visa-resource-name>)
              }
            }
            n138 = call "WT300 Get Data.vi"("error in (no error)"=w411, "VISA resource name"=w406) -> ("error out"=w410:errorcluster, "Yokogawa Data"=w409:string[][])  [unwired: 4 in, 4 out]
          }
          frame "WT210" {
            # "WT210 is now obsolete"
            n139 = Unbundle By Name(w419) -> ("Power.Yokogawa.WT210.Power VISA Yokogawa WT210"=w418:refnum<visa-resource-name>)
            n140 = call "WT210 Get Data.vi"("error in (no error)"=w422, "VISA resource name"=w418) -> ("error out"=w421:errorcluster, "Yokogawa Data"=w420:string[][])  [unwired: 4 in, 4 out]
          }
          frame "WT230" {
            n141 = Unbundle By Name(w425) -> ("Power.Yokogawa.WT210.Power VISA Yokogawa WT210"=w424:refnum<visa-resource-name>, "Power.Yokogawa.WT210.V Range (6: 600V)"=w423:i32)
            n142 = call "WT210 Get Data.vi"("Collect Element 3 Data"=TRUE, "error in (no error)"=w429, "Uthd:Element 1"=w423, "VISA resource name"=w424) -> ("error out"=w428:errorcluster, "Yokogawa Data"=w426:string[][])  [unwired: 2 in, 4 out]
          }
          frame "WT500" {
            # "WT500: I use this device for \nsplit phase. It will measure\neverything in the cluster"
            n143 = Unbundle By Name(w431) -> ("Power.Yokogawa.WT500.Power VISA Yokogawa WT500"=w430:refnum<visa-resource-name>)
            n144 = call "WT500 Get Power Data.vi"("Error In"=w434, "VISA resource name"=w430) -> ("Error Out"=w433:errorcluster, "Data Array"=w432:string[][])  [unwired: 3 in, 4 out]
          }
          frame "APLUS" {
            # "APLUS: This device does not \nsupport crest factors\nI only use for single phase 2W.\nI put zeros in all of the arrays \nassociated with split phase"
            n145 = Unbundle By Name(w437) -> ("Power.Aplus.Aplus IP Address"=w436:string, "Power.Aplus.Remote Port"=w435:i32)
            n146 = call "APLUS Camille Bauer Driver.vi"("error in (no error)"=w440, "Remote Port"=w435, "Remote IP Address"=w436) -> ("error out"=w439:errorcluster, "APLUS Data"=w438:string[][])  [unwired: 4 in, 3 out]
          }
          frame "Debug" {
            # "Debug Mode"
          }
        }
        n147 = Build Array (concatenate)(w398, w397) -> (w396:string[][])
        n148 = call <vilib>:"Add State(s) to Queue__jki_lib_state_machine.vi"("State(s) in (\"\")"=w405) -> ("States Out"=w404:string)  [unwired: 14 in]
        n149 = Bundle By Name(cluster=w399, "Total Array"=w396) -> (w403:T12)
      }
      frame "Disregard First Third" {
        # "Compute Column Averages"
        # "Disregard first third of test data"
        n150 = Unbundle By Name(w454) -> ("Standby Power Array.5 Min Data Array"=w448:dbl[][], "Loop Index"=w445:i32, "Total Array"=w444:string[][], "Standby Power In"=w451:T5)
        n151 = call "Standby Power Data Process.vi"("Loop Index"=w445, "Error In"=w452, "Standby Power In in"=w451, "Total Array Input"=w444, "Array DBL"=w448) -> ("Error Out"=w450:errorcluster, "Plot Data"=w446:string[][], "Average Data"=w443:string[][])  [unwired: 3 in, 1 out]
        n152 = call "UTILITY Create Plot Array.vi"("Error In"=w450, "Save Data"=w446, "Plot Array in"=w448) -> ("Error Out"=w449:errorcluster, "Plot Array out"=w447:dbl[][])  [unwired: 7 in]
        n153 = Bundle By Name(cluster=w454, "Standby Power Array.5 Min Data Array"=w447, "Total Array"=w443) -> (w453:T12)
        n154 = call <vilib>:"Add State(s) to Queue__jki_lib_state_machine.vi"("State(s) in (\"\")"=w456) -> ("States Out"=w455:string)  [unwired: 14 in]
      }
      frame "Collect for 15 Mins" {
        # "Compute Column Averages"
        n155 = Unbundle By Name(w465) -> ("Standby Power Array.15 Min Data Array"=w467:dbl[][], "Loop Index"=w460:i32, "Total Array"=w458:string[][], "Standby Power In"=w469:T5)
        n156 = call "Standby Power Data Process.vi"("Loop Index"=w460, "Error In"=w463, "Standby Power In in"=w469, "Total Array Input"=w458, "Array DBL"=w467) -> ("Error Out"=w468:errorcluster, "Standby Power In out"=w461:T5, "Plot Data"=w459:string[][], "Average Data"=w457:string[][])  [unwired: 3 in]
        n157 = call "UTILITY Create Plot Array.vi"("Error In"=w468, "Save Data"=w459, "Plot Array in"=w467) -> ("Error Out"=w462:errorcluster, "Plot Array out"=w466:dbl[][])  [unwired: 7 in]
        n158 = Bundle By Name(cluster=w465, "Standby Power Array.15 Min Data Array"=w466, "Standby Power In"=w461, "Total Array"=w457) -> (w464:T12)
        n159 = call <vilib>:"Add State(s) to Queue__jki_lib_state_machine.vi"("State(s) in (\"\")"=w471) -> ("States Out"=w470:string)  [unwired: 14 in]
      }
      frame "Show Data" {
        n160 = Unbundle By Name(w478) -> ("Current State"=w480:T11, "Total Array"=w473:string[][], "Save Data"=w475:string[][], "Write Header"=w476:bool)
        "Data" <- w473
        n161 = Unbundle By Name(w480) -> ("Part 1"=w472:bool)
        n162 = case shown="True" w472 {
          tunnel: w478 -> [w502 w504]
          tunnel: [w501 w503] -> w479
          frame False {
            n163 = Unbundle By Name(w502) -> ("Standby Power Array.15 Min Data Array"=w501:dbl[][])
          }
          frame True {
            n164 = Unbundle By Name(w504) -> ("Standby Power Array.5 Min Data Array"=w503:dbl[][])
          }
        }
        n165 = Transpose 2D Array(2D array=w473) -> (transposed array=w474:string[][])
        n166 = case shown="False" "Disable Plot" {
          tunnel: w474 -> [w511 _]
          tunnel: w479 -> [w508 _]
          frame False {
            n167 = call "UTILITY MultiPlot.vi"("Y-Axis-2"="Y-Axis-2", "Y-Axis-1"="Y-Axis-1", "X-Axis"="X-Axis", "Save Data"=w511, "Plot Array"=w508) -> ("Plot Cluster"=w510:T2)  [unwired: 5 in, 1 out]
            n168 = case shown="False" "Pause Graph" {
              tunnel: w510 -> [w512 _]
              frame False {
                "XY Graph" <- w512
              }
              frame True {
              }
            }
          }
          frame True {
          }
        }
        n169 = case shown="False" w472 {
          tunnel: w478 -> [w491 w500]
          tunnel: [w490 w500] -> w477
          tunnel: w476 -> [w489 _]
          tunnel: w475 -> [w487 _]
          tunnel: w474 -> [w486 _]
          frame False {
            n170 = case shown="False" w489 {
              tunnel: w487 -> [w496 w499]
              tunnel: [w492 w498] -> w488
              tunnel: w486 -> [w494 w497]
              frame False {
                n171 = Index Array(array=w494, index (row)=1) -> (element=w493:string[])  [unwired: 1 in]
                n172 = Build Array (concatenate)(w496, w493) -> (w492:string[][])
              }
              frame True {
                n173 = Build Array (concatenate)(w499, w497) -> (w498:string[][])
              }
            }
            n174 = Bundle By Name(cluster=w491, "Save Data"=w488, "Write Header"=FALSE) -> (w490:T12)
          }
          frame True {
          }
        }
        n175 = call <vilib>:"Add State(s) to Queue__jki_lib_state_machine.vi"("State(s) in (\"\")"=w484) -> ("States Out"=w483:string)  [unwired: 14 in]
      }
      frame "Error Check" {
        n176 = Unbundle By Name(w519) -> ("Standby Power In"=w516:T5, "Power"=w514:T3)
        n177 = local read "Elapsed Time."() -> (w515:dbl)
        n178 = local read "User Notice"() -> (w513:string)
        n179 = call "Generate Error.vi"("Elapsed Time (s)"=w515, "error in (no error)"=w520, "Power"=w514, "Message Input"=w513, "Standby Power In"=w516) -> ("error out"=w523:errorcluster, "Error?"=w517:bool, "Message Out"=w521:string, "States"=w522:string)  [unwired: 3 in]
        n180 = local write "User Notice"(w521) -> ()
        n181 = Bundle By Name(cluster=w519, "Error?"=w517) -> (w518:T12)
        n182 = call <vilib>:"Add State(s) to Queue__jki_lib_state_machine.vi"("State(s) in Front (\"\")"=w522, "State(s) in (\"\")"=w525) -> ("States Out"=w524:string)  [unwired: 13 in]
      }
      frame "----Data Processing----" {
      }
      frame "Data Process" {
        n183 = Unbundle By Name(w534) -> ("Standby Power Array"=w537:T10, "Power"=w538:T3, "Standby Power In"=w539:T5, "Data Process Timer Reset"=w532:bool, "Loop Index"=w540:i32, "Total Array"=w529:string[][])
        n184 = call "Standby Power Calculate Slope.vi"("Standby Power Array"=w537, "Total Array"=w529, "Power"=w538, "Error In"=w542, "Loop Index"=w540, "Timer Reset"=w532, "Standby Power In"=w539) -> ("Error Out"=w541:errorcluster, "Loop Index Output"=w535:i32, "Test Complete"=w536:bool, "Standby Power Out"=w530:T5)  [unwired: 1 in]
        n185 = case shown="True" w536 {
          tunnel: ["" "Final Harmonics\nCreate Output Data\nReset Power Meter\nMacro: Exit"] -> w543
          frame False {
          }
          frame True {
          }
        }
        n186 = flat-sequence {
          tunnel: w535 -> [w549]
          tunnel: w534 -> [w548]
          tunnel: [w547] -> w533
          tunnel: w530 -> [w545]
          frame #0 {
            n187 = Bundle By Name(cluster=w548, "Standby Power In"=w545, "Loop Index"=w549, "Data Process Timer Reset"=FALSE) -> (w547:T12)
          }
        }
        n188 = call <vilib>:"Add State(s) to Queue__jki_lib_state_machine.vi"("State(s) in Front (\"\")"=w543, "State(s) in (\"\")"=w531) -> ("States Out"=w544:string)  [unwired: 13 in]
      }
      frame "---Add Final Information---" {
        n189 = call <vilib>:"Add State(s) to Queue__jki_lib_state_machine.vi"("State(s) in (\"\")"=w554) -> ("States Out"=w555:string)  [unwired: 14 in]
      }
      frame "Final Harmonics" {
        n190 = Unbundle By Name(w559) -> ("Power Analyzer"=w563:T4, "Power"=w560:T3)
        n191 = case shown="\"WT300\", Default" w563 {
          tunnel: [w567 w571 w577 w583 w593] -> w561
          tunnel: [w566 "" w580 "" w592] -> w556
          tunnel: w562 -> [w567 w572 w578 w584 w593]
          tunnel: [w566 w570 w579 w588 w592] -> w557
          tunnel: w560 -> [_ w569 w575 w587 _]
          frame "WT300", Default {
            w566 = "WT333"
          }
          frame "WT210", "WT230" {
            n192 = Unbundle By Name(w569) -> ("Yokogawa.WT210.Power VISA Yokogawa WT210"=w568:refnum<visa-resource-name>)
            n193 = call "WT200 GET Harmonics.vi"("error in (no error)"=w572, "VISA Refnum in"=w568) -> ("error out"=w571:errorcluster, "Final Harmonic Content U1"=w570:string)  [unwired: 6 in, 2 out]
          }
          frame "WT500" {
            n194 = Unbundle By Name(w575) -> ("Yokogawa.WT500.Power VISA Yokogawa WT500"=w574:refnum<visa-resource-name>)
            n195 = call "WT500 Get Power Data.vi"("Error In"=w578, "VISA resource name"=w574) -> ("Error Out"=w577:errorcluster, "Power Data Out"=w576:T14)  [unwired: 3 in, 4 out]
            n196 = Unbundle By Name(w576) -> ("Voltage Harmonic (%):Element 1"=w582:dbl, "Voltage Harmonic (%):Element 2"=w581:dbl)
            n197 = Number To Fractional String(number=w582) -> (F-format string=w579:string)  [unwired: 3 in]
            n198 = Number To Fractional String(number=w581) -> (F-format string=w580:string)  [unwired: 3 in]
          }
          frame "APLUS" {
            n199 = Unbundle By Name(w587) -> ("Aplus.Aplus IP Address"=w586:string, "Aplus.Remote Port"=w585:i32)
            n200 = call "APLUS Camille Bauer Driver.vi"("error in (no error)"=w584, "Remote Port"=w585, "Remote IP Address"=w586) -> ("error out"=w583:errorcluster, "Power Data"=w591:T14)  [unwired: 4 in, 3 out]
            n201 = Unbundle By Name(w591) -> ("Voltage Harmonic (%):Element 1"=w589:dbl)
            n202 = Number To Fractional String(number=w589) -> (F-format string=w588:string)  [unwired: 3 in]
          }
          frame "Debug" {
            w592 = "Debug"
          }
        }
        n203 = Bundle By Name(cluster=w559, "Standby Power In.Final Harmonics-U1 (%)"=w557, "Standby Power In.Final Harmonics-U2 (%)"=w556) -> (w558:T12)
        n204 = call <vilib>:"Add State(s) to Queue__jki_lib_state_machine.vi"("State(s) in (\"\")"=w564) -> ("States Out"=w565:string)  [unwired: 14 in]
      }
      frame "Create Output Data" {
        # "Add final harmonics to title"
        # "Compile Data Export Sheet"
        n205 = Unbundle By Name(w606) -> ("Error?"=w599:bool, "Header File"=w604:string[][], "Standby Power In"=w602:T5, "Appliance Common"=w594:T1, "Save Data"=w601:string[][])
        n206 = local read "Elapsed Time."() -> (w603:dbl)
        n207 = call "Final Harmonics.vi"("Header File Input"=w604, "Error Output?"=w599, "Standby Power In 2"=w602, "Elapsed Time."=w603, "Appliance Common"=w594, "error in (no error)"=w605) -> ("Header File Output"=w600:string[][], "Standby Power Out"=w598:T5, "error out"=w608:errorcluster)  [unwired: 7 in]
        n208 = Bundle By Name(cluster=w606, "Standby Power In"=w598) -> (w597:T12)
        n209 = Build Array (concatenate)(w600, w601) -> (w595:string[][])
        n210 = Bundle By Name(cluster=w597, "Standby Power In.Standby Power Spreadsheet"=w595) -> (w596:T12)
        n211 = local write "User Notice"("Creating Output File...") -> ()
        n212 = call <vilib>:"Add State(s) to Queue__jki_lib_state_machine.vi"("State(s) in (\"\")"=w607) -> ("States Out"=w610:string)  [unwired: 14 in]
      }
    }
    n213 = case shown="True" "Debug?" {
      tunnel: w15 -> [_ w29]
      tunnel: w13 -> [w26 w28]
      tunnel: [w26 w27] -> w14
      frame False {
      }
      frame True {
        n214 = Build Array (concatenate)(w28, w29) -> (w27:string[])
        "Debug State" <- w27
      }
    }
  }
  "Error Out" <- w5
  n215 = Unbundle By Name(w3) -> ("Standby Power In"=→"Standby Power Out":T5)
